vi "GINKGO - MTMP - 20180214B.vi"() -> ()   [LabVIEW 2015]
uses:
  <vilib>/rvi/interface/nirviMethod/nirviMethod.xnode
  <vilib>/rvi/interface/nirviCloseFPGA/nirviCloseFPGA.xnode
  <vilib>/rvi/interface/nirviReadWriteControl/nirviReadWriteControl.xnode
  <vilib>/rvi/interface/nirviOpenFPGA/nirviOpenFPGA.xnode
  <vilib>/rvi/interface/Simulation/niFpgaSimulationCallBeginRW.vi
  <vilib>/rvi/errors/niLvFpgaAdjustHostInterfaceError.vi
  <vilib>/rvi/errors/niLvFpgaMergeErrorWithErrorCode.vi
  <vilib>/FPGAPlugInAG/Dynamic/niLvFpga_Abort_Dynamic.vi
  <vilib>/FPGAPlugInAG/Dynamic/niLvFpga_Reset_Dynamic.vi
  <vilib>/FPGAPlugInAG/Dynamic/niLvFpga_Run_Dynamic.vi
  NiFpgaLv.dll
  <vilib>/Utility/error.llb/Error Cluster From Error Code.vi
  <vilib>/FPGAPlugInAG/Dynamic/niLvFpga_Close_Dynamic.vi
  <vilib>/FPGAPlugInAG/Dynamic/niLvFpga_ReadFifo_Dynamic.vi
  <vilib>/rvi/interface/common/dynamic/niFpgaDynamicAddResources.vi
  <vilib>/FPGAPlugInAG/Dynamic/niLvFpga_StopFifo_Dynamic.vi
  Controls/Save picture camera.vi
  <vilib>/vision/NI_Vision_Development_Module.lvlib
  Global Variable/GV_Z axis.vi
  Global Variable/GV_Lock State.vi
  <vilib>/FPGAPlugInAG/Dynamic/niLvFpga_WriteFifo_Dynamic.vi
  <vilib>/FPGAPlugInAG/Dynamic/niLvFpga_ConfigureFifo_Dynamic.vi
  <vilib>/FPGAPlugInAG/Dynamic/niLvFpga_StartFifo_Dynamic.vi
  FPGA Bitfiles/GINKGO-MTPM_7854R_FPGAControl5_d88-Mrxru6Q.lvbitx
  FPGA/FPGA Control.vi
  <vilib>/FPGAPlugInAG/PXI-7854R/niLvFpga_Open_PXI-7854R.vi
  FPGA Bitfiles/GINKGO-MTPM_7975R_FPGA796xR_a2zTekeNlbw.lvbitx
  FPGA/FPGA 796xR.vi
  <vilib>/FPGAPlugInAG/PXIe-7975R/niLvFpga_Open_PXIe-7975R.vi
  FPGA Bitfiles/GINKGO-MTPM_7853R_FPGAControl5_UMX-AIE6YDk.lvbitx
  <vilib>/FPGAPlugInAG/PXI-7853R/niLvFpga_Open_PXI-7853R.vi
  FPGA Bitfiles/GINKGO-MTPM_7961R_FPGA796xR2_HwVDrqHPH4U.lvbitx
  <vilib>/FPGAPlugInAG/PXIe-7961R/niLvFpga_Open_PXIe-7961R.vi
panel:
  out "波形图表":sgl(graph)=113.25391
  in  "ROI Statistic":bool=TRUE
  out "Mean Value":sgl=113.25391
  out "Variation":sgl=54.35391
  out "Minimal":sgl=32720.0
  out "Maximal":sgl=33176.0
  out "Power Stop":bool=TRUE
  in  "Rolling Queue Flag":bool=TRUE
  out "Total Data Out":u16=13612
  in  "Acq. Start":u16=38 caption="Phase" max=6000 step=1
  in  "Real Back Period":u16=5 min=1
  out "实际深度":u32=8388608
  in  "Map Max.":i32=10000 caption="Max."
  in  "Map Min.":i32=-500 caption="Min."
  out "Scale Value":dbl=0.1 caption="X"
  out "Total Frames":u16=16553
  in  "Max. Min.":cluster{i32, i32}(slide)={429, -176} scale=-500.0..10000.0
  in  "16-bit Display Method":u32(ring)=14 caption="Display Method" items=["Full Dynamic"=12, "Given Range"=14]
  in  "Rolling Average":dbl=2.0 min=1.0 step=1.0
  in  "Rolling":bool=TRUE
  out "User Define Phase":u32=746
  out "Image":T1(plugin-control)
  in  "Controls":T2(tab)
  in  "Start Device":bool
  in  "PMT Shutter Pow.":bool
  out "Overload Dis.":bool=TRUE
  in  "Pulse Number":enum16{"SP", "DP"}(ring)
  in  "Mems Enable":bool
  out "中心偏移":i32
  in  "互相关点数":i32=5
  in  "Calculate Phase shift":bool
  in  "Wave":enum16{"Triangle", "Sine", "Ramp"}(ring)=enum."Sine"
  in  "Interval Dis.":sgl=0.00049965957 min=-10 max=50 format="%.4f"
  in  "stop z stage":bool
  in  "5V":bool
  in  "Voltage Level":dbl=15.0 format="%#.3p"
  in  "Voltage Level 2":dbl=-15.0 caption="Voltage Level" format="%#.3p"
  in  "Source:Output Enabled":bool
  out "Voltage Measurement 2":dbl=-0.0001217159676001422 caption="Voltage Measurement"
  out "Compliance/Limit Reached 2":bool caption="Compliance/Limit Reached"
  out "Voltage Measurement":i8
  out "Compliance/Limit Reached":bool
  in  "MEMS SLOW":dbl(slide)=240000.0 caption="Slow" min=0.0 max=1000000.0 step=100.0 scale=0.0..300000.0 scale format="%#_6p"
  in  "MEMS FAST":dbl(slide) caption="Fast" min=0.0 max=1000000.0 step=100.0 scale=0.0..300000.0 scale format="%#_6p"
  out "Stimulate Time Dis.":u32
  in  "Stimulate Value":dbl=5.0 min=-10.0 max=10.0 format="%#_3f"
  in  "Stimulate Time":u32=500
  out "Stimulate Interval Time":dbl=1.9692307692307693
  in  "Stimulate Interval":u32=10
  in  "Stimulate Enable":bool caption="V.S."
  out "Frame Befor Time":dbl=845778175.0153847
  out "Frame Number":u32=4294967295
  in  "Frames Befor Stimulate":u32
  out "Acq. Sample Rate":dbl=120000000.0 caption="Sanple Rate Divider" format="%#_6p"
  in  "Microscope":enum16{"Miniature", "Benchtop"}(ring)
  in  "Line":u32(ring)=512 caption="Y" items=["8"=8, "16"=16, "32"=32, "64"=64, "128"=128, "256"=256, "512"=512, "1024"=1024, "2048"=2048]
  in  "X Offset":dbl caption="X" format="%#_3f"
  in  "Y Offset":dbl caption="Y" min=-10.0 max=10.0 format="%#_3f"
  in  "X Frequency":dbl(slide)=2600.0 caption="Speed" min=50.0 max=10000.0 step=1.0 scale=0.0..5000.0
  in  "Laser Intensity":dbl(slide)=2.0786516853932584 max=10.0 scale=0.0..5.0
  in  "Phase Shift":u32(slide)=752 caption="Phase" max=15000 step=2 scale=0.0..15000.0
  in  "Point":bool
  in  "PMT1 Sensitivity":dbl(slide)=0.5 min=0.0 max=0.95 step=0.05 scale=0.0..0.95 scale format="%#_3f"
  in  "PMT1 Enable":bool=TRUE
  out "Pixel Dwell":dbl=0.2988 format="%#_3g"
  out "Actual Positon":sgl=11.119017
  out "Actual Laser Intensity":dbl(knob)=0.69488525390625 scale=-10.0..1.0
  in  "PMT2 Switch":bool
  in  "PMT2 Sensitivity":dbl(slide)=0.45 min=0.0 max=0.95 step=0.05 scale=0.0..0.95 scale format="%#_3f"
  in  "File Name":string
  in  "Scale":bool
  in  "XY Home":bool
  in  "XY UP":bool
  in  "XY DOWN":bool
  in  "XY LEFT":bool
  in  "XY RIGHT":bool
  in  "Stop":bool=TRUE
  in  "LIVE":bool
  in  "Save":bool
  in  "Z-Stack":bool
  in  "Pixel/Line":u16(ring)=512 caption="X" items=["8"=8, "16"=16, "32"=32, "64"=64, "128"=128, "256"=256, "512"=512, "1024"=1024, "2048"=2048]
  in  "Gain":enum16{"0dB", "6dB", "12dB"}(ring)
  in  "Coulple":enum16{"AC", "DC"}(ring)=enum."DC"
  in  "Path":path=path "C:/Users/TVS001/Desktop/DATA/20180207/13-zz-gcamp" caption="Images Folder"
  out "Save Frames Dis.":u16=1000
  in  "Save Frames":u16=1000
  in  "ZOOM":u16(ring)=2 items=["User Define", "1X", "1.5X", "2X", "2.5X", "3X", "3.5X", "4X", "4.5X", "5X", "6X"]
  in  "Scan Mode":enum16{"Normal", "Line Scan", "Random Access"}(ring)
  in  "Y Amplitude":dbl=0.6 caption="Y" min=-10.0 max=18.0 format="%0.2p"
  in  "X Amplitude":dbl=0.6 caption="X" min=-10.0 max=18.0 format="%.2p"
  in  "Add Phase":bool
  in  "Move":bool=TRUE
  out "Frame Rate":dbl=5.078125 format="%#_3g"
  out "Ready":u8(slide)=10 scale=0.0..10.0
  in  "Z":bool
  out "Position":sgl=-5.9652176 format="%#_6f"
  in  "Set Zero":bool caption="空白按钮"
  in  "Reset Zero":bool caption="空白按钮"
  in  "Home Z":bool
  in  "Abs. Go":bool
  in  "Abs Pos X":sgl min=-10 max=360 format="%.6f"
  in  "Z Up":bool
  in  "Z Down":bool
  in  "Jog":sgl=0.0005 caption="Z" min=0 max=50 step=0.0001 format="%.4f"
  in  "Frames/Slice":u16=5
  in  "Slices":u16=87
  out "End Dis.":sgl=0.043470383 format="%#_6f"
  out "Start Dis.":sgl format="%#_6f"
  in  "End":bool
  in  "Start":bool
  in  "Restart":bool
  in  "Interval Time":u32=150
  in  "Zoom Standard":dbl[][](array[numeric])=[[10.0, 10.0, 11251.0], [6.66, 6.66, 10603.0], [5.0, 5.0, 10394.0], [4.0, 4.0, 10394.0], [3.34, 3.34, 8602.0], [2.86, 2.86, 10394.0], [2.5, 2.5, 10394.0], [2.222, 2.222, 10394.0], [1.3, 1.3, 8294.0], [0.6, 0.6, 8296.0]]
  in  "Zoom Miniature":dbl[][](array[numeric])=[[14.0, 8.0, 738.0], [12.0, 7.0, 746.0], [9.0, 6.0, 752.0], [7.2, 5.6, 754.0], [5.0, 4.0, 738.0], [5.14, 4.0, 846.0], [4.0, 3.0, 744.0], [3.6, 2.0, 840.0], [3.2, 2.3, 754.0], [3.0, 2.33, 740.0]]
  out "Test Point2":u32
  out "Test Point 3":u32=143394
  out "Test Point":u32
  out "Point/Pixel":i32=36
  in  "Focus Flag":bool
  out "Queue Number":i32=2
  out "Initial Z":bool
  out "Initialization Done":bool=TRUE
  in  "Start Control":bool
  out "Memory":i32(slide) scale=0.0..5000.0
  in  "Resource Name":refnum<k15>="PXI1Slot6"
  in  "Channel Name":string="1" caption="Channel Name 1"
  in  "Current Limit":dbl=0.5 format="%.3p"
  in  "Voltage Level Range":dbl=20.0 format="%.5p"
  in  "Current Limit Range":dbl=1.0 format="%.3p"
  in  "Source Delay (Sec)":dbl=0.1 format="%.3p"
  in  "Channel Name 2":string="2"
  out "Current Measurement 2":dbl=-3.1048749529460624e-06 caption="Current Measurement"
  out "Current Measurement":i16
  out "Actual DDS Ticks":u32=1
  out "Actual DDS Sample Freq":u32=279173
  in  "OUTPUT Value Ticks":u32=44
  in  "DDS Ticks":u32=1
  out "Actual OUTPUT Value Ticks":u32=44
  in  "Random 1D Array":fxp<+/-,32,16>[](array[numeric]) format="%.21g"
  in  "MG17Motor Z":refnum<k7>(container)
  out "Acq. Point Dis.":u16=32
  in  "Divide":enum16{"120M", "60M", "30M", "15M", "7.5M"}(ring)
  out "Nonlinear Acq.":bool=TRUE
  in  "Adapter Module User Data 1":u8
  in  "Adapter Module User Data 0":u8
  in  "Adapter Module User Command":u8=3
  in  "Apply":bool
  in  "HWSerialNum":i32=49871607
  in  "Set Large Scale":dbl=0.5 caption="X"
  in  "Set Small Scale":dbl=0.1 caption="X"
  in  "Set Zero Value":sgl format="%#_6f"
  in  "Fill Fraction":dbl=0.8 min=0.1 max=6.0 step=0.01
  in  "Back Period":u16=5 min=1
  in  "Initial Benchtop Speed":dbl=500.0 caption="Speed" min=50.0 max=10000.0 step=1.0
  in  "Initial Miniature Speed":dbl=2600.0 caption="Speed" min=50.0 max=10000.0 step=1.0
  out "Acq.Point Array":u16[](graph)=[38, 38, 38, 37, 37, 37, 37, 36, 36, 36, 36, 36, 35, 35, 35, 35, 35, 34, 34, 34, 34, 34, 34, 33, 33, 33, 33, 33, 33, 32, 32, 32, 32, 32, 32, 32, 32, 31, 31, 31, 31, 31, 31, 31, 31, 30, 30, 30, 30, 30, 30, 30, 30, 30, 30, 29, 29, 29, 29, 29, 29, 29, 29, 29, 29, 29, 28, 28, 28, 28, 28, 28, 28, 28, 28, 28, 28, 28, 28, 28, 27, 27, 27, 27, 27, 27, 27, 27, 27, 27, 27, 27, 27, 27, 27, 27, 26, 26, 26, 26, 26, 26, 26, 26, 26, 26, 26, 26, 26, 26, 26, 26, 26, 26, 26, 26, 26, 25, 25, 25, 25, 25, 25, 25, 25, 25, 25, 25, 25, 25, 25, 25, 25, 25, 25, 25, 25, 25, 25, 25, 25, 25, 25, 25, 24, 24, 24, 24, 24, 24, 24, 24, 24, 24, 24, 24, 24, 24, 24, 24, 24, 24, 24, 24, 24, 24, 24, 24, 24, 24, 24, 24, 24, 24, 24, 24, 24, 24, 24, 24, 24, 24, 24, 24, 24, 24, 24, 23, 23, 23, 23, 23, 23, 23, 23, 23, 23, 23, 23, 23, 23, 23, 23, 23, 23, 23, 23, 23, 23, 23, 23, 23, 23, 23, 23, 23, 23, 23, 23, 23, 23, 23, 23, 23, 23, 23, 23, 23, 23, 23, 23, 23, 23, 23, 23, 23, 23, 23, 23, 23, 23, 23, 23, 23, 23, 23, 23, 23, 23, 23, 23, 23, 23, 23, 23, 23, 23, 23, 23, 23, 23, 23, 23, 23, 23, 23, 23, 23, 23, 23, 23, 23, 23, 23, 23, 23, 23, 23, 23, 23, 23, 23, 23, 23, 23, 23, 23, 23, 23, 23, 23, 23, 23, 23, 23, 23, 23, 23, 23, 23, 23, 23, 23, 23, 23, 23, 23, 23, 23, 23, 23, 23, 23, 23, 23, 23, 23, 23, 23, 23, 23, 23, 23, 23, 23, 24, 24, 24, 24, 24, 24, 24, 24, 24, 24, 24, 24, 24, 24, 24, 24, 24, 24, 24, 24, 24, 24, 24, 24, 24, 24, 24, 24, 24, 24, 24, 24, 24, 24, 24, 24, 24, 24, 24, 24, 24, 24, 24, 25, 25, 25, 25, 25, 25, 25, 25, 25, 25, 25, 25, 25, 25, 25, 25, 25, 25, 25, 25, 25, 25, 25, 25, 25, 25, 25, 26, 26, 26, 26, 26, 26, 26, 26, 26, 26, 26, 26, 26, 26, 26, 26, 26, 26, 26, 26, 26, 27, 27, 27, 27, 27, 27, 27, 27, 27, 27, 27, 27, 27, 27, 27, 27, 28, 28, 28, 28, 28, 28, 28, 28, 28, 28, 28, 28, 28, 28, 29, 29, 29, 29, 29, 29, 29, 29, 29, 29, 29, 30, 30, 30, 30, 30, 30, 30, 30, 30, 30, 31, 31, 31, 31, 31, 31, 31, 31, 32, 32, 32, 32, 32, 32, 32, 32, 33, 33, 33, 33, 33, 33, 34, 34, 34, 34, 34, 34, 35, 35, 35, 35, 35, 36, 36, 36, 36, 36, 37, 37, 37, 37, 38, 38, 38]
  out "Init Data Out":u16[](array[numeric])=[38, 38, 38, 37, 37, 37, 37, 36, 36, 36, 36, 36, 35, 35, 35, 35, 35, 34, 34, 34, 34, 34, 34, 33, 33, 33, 33, 33, 33, 32, 32, 32, 32, 32, 32, 32, 32, 31, 31, 31, 31, 31, 31, 31, 31, 30, 30, 30, 30, 30, 30, 30, 30, 30, 30, 29, 29, 29, 29, 29, 29, 29, 29, 29, 29, 29, 28, 28, 28, 28, 28, 28, 28, 28, 28, 28, 28, 28, 28, 28, 27, 27, 27, 27, 27, 27, 27, 27, 27, 27, 27, 27, 27, 27, 27, 27, 26, 26, 26, 26, 26, 26, 26, 26, 26, 26, 26, 26, 26, 26, 26, 26, 26, 26, 26, 26, 26, 25, 25, 25, 25, 25, 25, 25, 25, 25, 25, 25, 25, 25, 25, 25, 25, 25, 25, 25, 25, 25, 25, 25, 25, 25, 25, 25, 24, 24, 24, 24, 24, 24, 24, 24, 24, 24, 24, 24, 24, 24, 24, 24, 24, 24, 24, 24, 24, 24, 24, 24, 24, 24, 24, 24, 24, 24, 24, 24, 24, 24, 24, 24, 24, 24, 24, 24, 24, 24, 24, 23, 23, 23, 23, 23, 23, 23, 23, 23, 23, 23, 23, 23, 23, 23, 23, 23, 23, 23, 23, 23, 23, 23, 23, 23, 23, 23, 23, 23, 23, 23, 23, 23, 23, 23, 23, 23, 23, 23, 23, 23, 23, 23, 23, 23, 23, 23, 23, 23, 23, 23, 23, 23, 23, 23, 23, 23, 23, 23, 23, 23, 23, 23, 23, 23, 23, 23, 23, 23, 23, 23, 23, 23, 23, 23, 23, 23, 23, 23, 23, 23, 23, 23, 23, 23, 23, 23, 23, 23, 23, 23, 23, 23, 23, 23, 23, 23, 23, 23, 23, 23, 23, 23, 23, 23, 23, 23, 23, 23, 23, 23, 23, 23, 23, 23, 23, 23, 23, 23, 23, 23, 23, 23, 23, 23, 23, 23, 23, 23, 23, 23, 23, 23, 23, 23, 23, 23, 23, 24, 24, 24, 24, 24, 24, 24, 24, 24, 24, 24, 24, 24, 24, 24, 24, 24, 24, 24, 24, 24, 24, 24, 24, 24, 24, 24, 24, 24, 24, 24, 24, 24, 24, 24, 24, 24, 24, 24, 24, 24, 24, 24, 25, 25, 25, 25, 25, 25, 25, 25, 25, 25, 25, 25, 25, 25, 25, 25, 25, 25, 25, 25, 25, 25, 25, 25, 25, 25, 25, 26, 26, 26, 26, 26, 26, 26, 26, 26, 26, 26, 26, 26, 26, 26, 26, 26, 26, 26, 26, 26, 27, 27, 27, 27, 27, 27, 27, 27, 27, 27, 27, 27, 27, 27, 27, 27, 28, 28, 28, 28, 28, 28, 28, 28, 28, 28, 28, 28, 28, 28, 29, 29, 29, 29, 29, 29, 29, 29, 29, 29, 29, 30, 30, 30, 30, 30, 30, 30, 30, 30, 30, 31, 31, 31, 31, 31, 31, 31, 31, 32, 32, 32, 32, 32, 32, 32, 32, 33, 33, 33, 33, 33, 33, 34, 34, 34, 34, 34, 34, 35, 35, 35, 35, 35, 36, 36, 36, 36, 36, 37, 37, 37, 37, 38, 38, 38]
  out "x amp. new":dbl
  out "y amp. new":dbl
  in  "Add Random Access":bool
  out "x offset new":i16=-7638
  out "y offset new":i16=-4030
  in  "All Random Array":fxp<+/-,32,16>[][](array[numeric])
  in  "Clear Array":bool
  out "Random Phase":u32=12 caption="Phase" max=6000 step=1
  # "File Name"
  # "File Path"
  # "Save Frames"
  # "Microscope"
  # "Scan Mode"
  # "PMT1"
  # "PMT2"
  # "Frame Size"
  # "Gain"
  # "Scan Speed"
  # "Hz"
  # "V"
  # "V"
  # "Rate"
  # "Frame Rate"
  # "μs"
  # "Hz"
  # "Pixel Dwell"
  # "XY"
  # "Z"
  # "Zoom"
  # "Point"
  # "Amplitude"
  # "V"
  # "V"
  # "Phase"
  # "Laser"
  # "Intensity Map"
  # "Recent Z"
  # "Frames Before"
  # "s"
  # "Stimulate Interval"
  # "s"
  # "ms"
  # "Stimulate Time"
  # "V"
  # "Stimulate Intensity"
  # "Mode Switch"
  # "MEMS Filter"
  # "Acquisition Mode"
  # "Image Settings"
  # "Magnification"
  # "Save Settings"
  # "Position Settings"
  # "Detection Settings"
  # "Z-scan Settings"
  # "Vision Stimulate Settings"
  # "X"
  # "Y"
  # "Phase"
  # "1X"
  # "1.5X"
  # "2X"
  # "2.5X"
  # "3X"
  # "3.5X"
  # "4X"
  # "4.5X"
  # "5X"
  # "6X"
  # "X"
  # "Y"
  # "Phase"
  # "1X"
  # "1.5X"
  # "2X"
  # "2.5X"
  # "3X"
  # "3.5X"
  # "4X"
  # "4.5X"
  # "5X"
  # "6X"
  # "40859011"
  # "83856379"
  # "AO0 -- X-Miniature  \nAO1 -- Y-Miniature\nAO2 -- Laser Intensity\nAO3 -- PMT1\nAO4 -- PMT2 \nAO5 -- \nAO6 -- X-Benchtop\nAO7 -- Y-Benchtop\n\nAI0  -- Actual Laser Intensity"
  # "DIO0 -- Acqusition  \nDIO1 -- VSYNC\nDIO2 -- HSYNC \nDIO3 -- Laser Shutter\nDIO4 -- MEMS FAST Filter\nDIO5 -- MEMS SLOW Filter\nDIO6 -- PMT Shutter\nDIO7 -- PMT Shutter Pow.\nDIO8 -- Shock Detection \nDIO9 -- Foot-plate LIVE Detection"
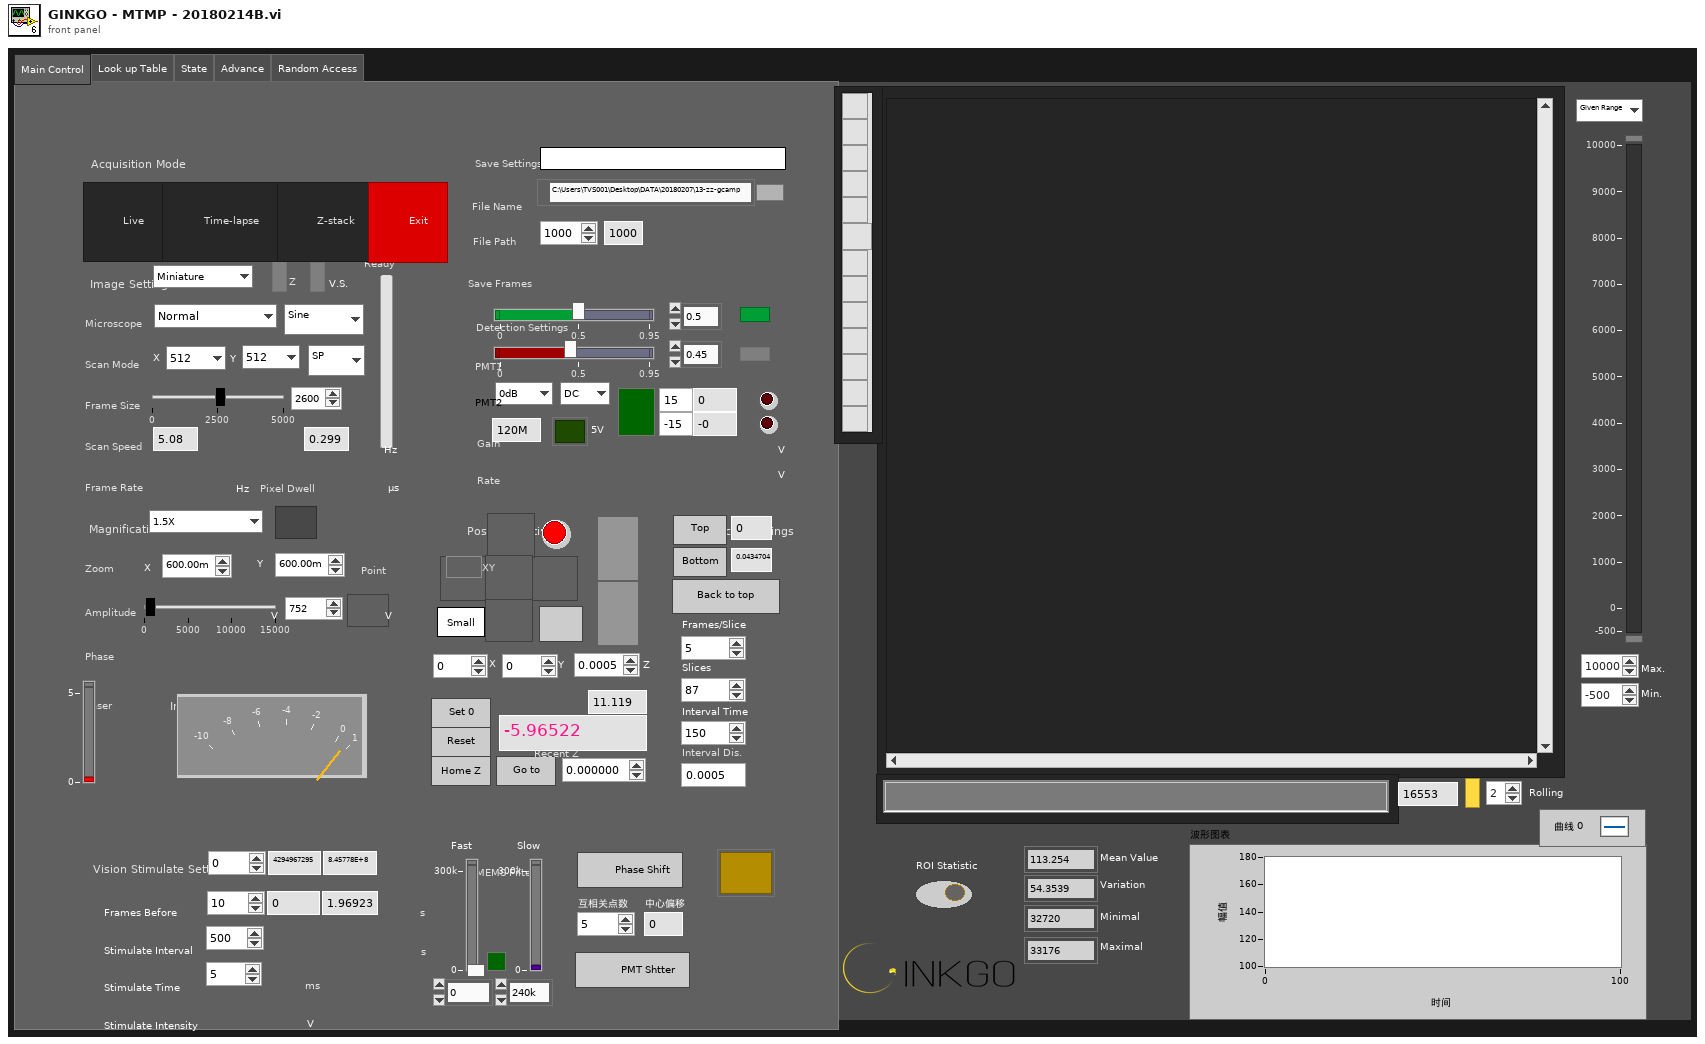
[diagram p1: front panel]
types:
  T1 = typedef "IMAQ Image.ctl" = refnum<image>
  T2 = enum32{"Main Control", "Look up Table", "State", "Advance", "Random Access"}
  T3 = typedef "Image Type" = u32
  T4 = enum8{"Enabled", "Disabled", "Disabled and Grayed Out"}
  T5 = cluster{"Global Rectangle":i32[], "Contours":cluster{"Contour Type":u32, "ROI Type":u32, "Points":i32[]}[]}
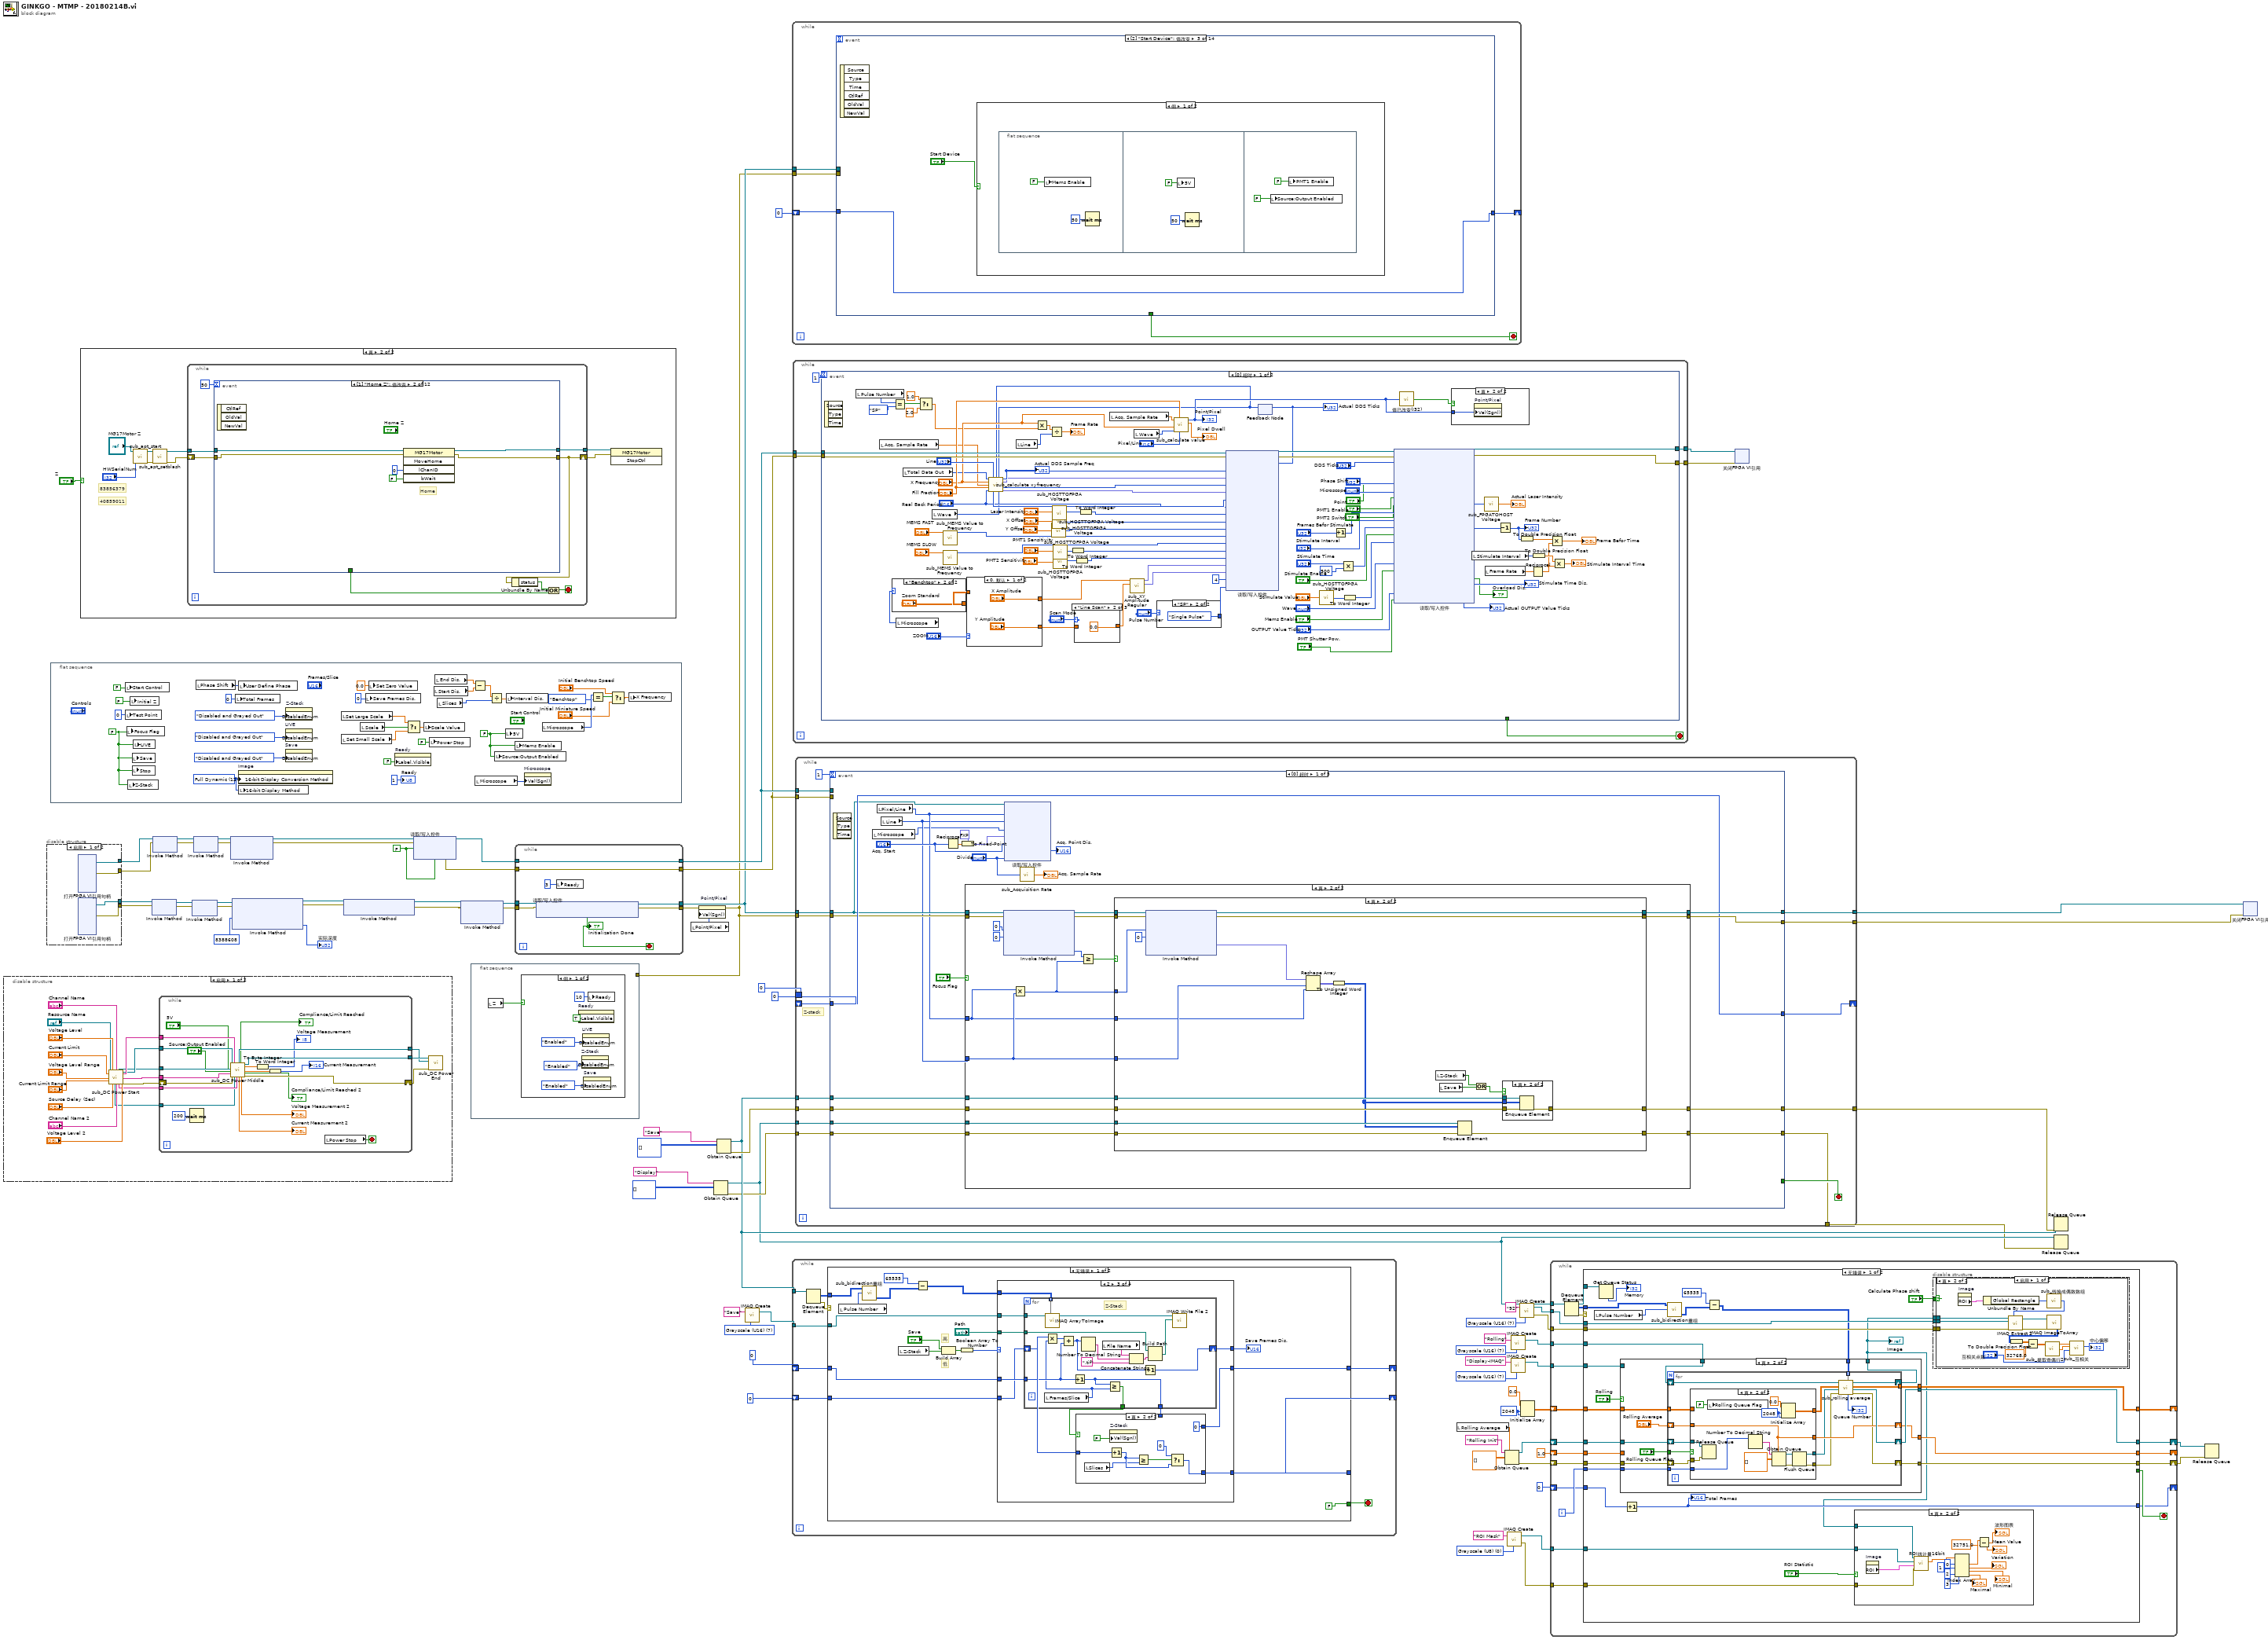
[diagram p0: block diagram]
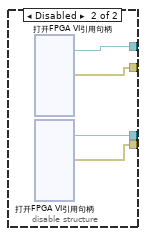
[diagram p2: hidden frame]
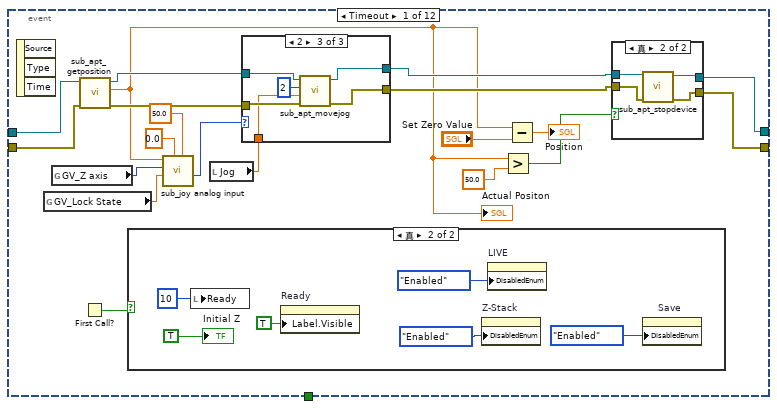
[diagram p4: hidden frame]
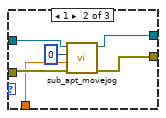
[diagram p6: hidden frame]
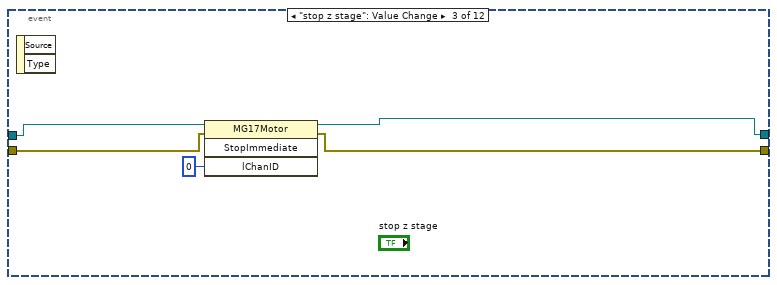
[diagram p9: hidden frame]
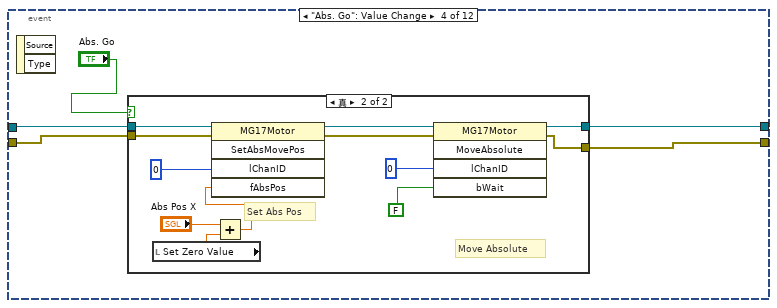
[diagram p10: hidden frame]
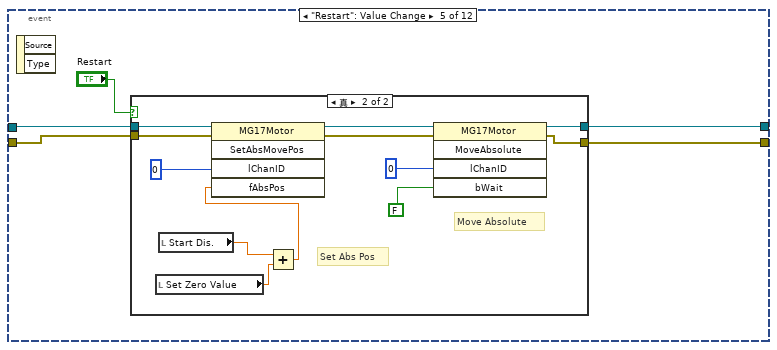
[diagram p12: hidden frame]
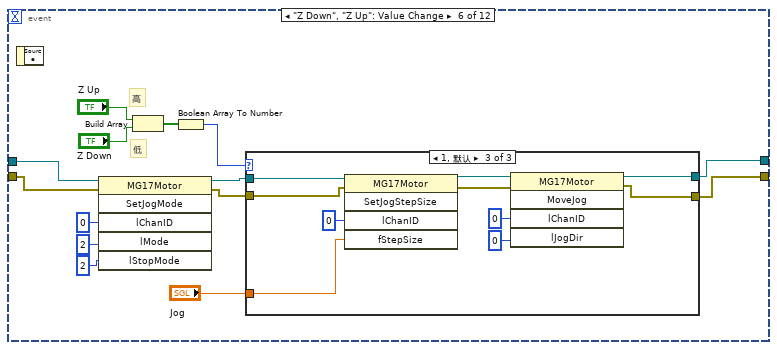
[diagram p14: hidden frame]
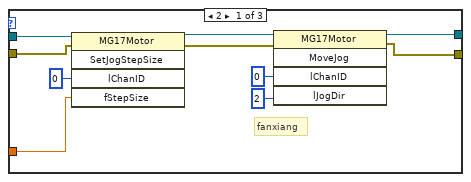
[diagram p15: hidden frame]
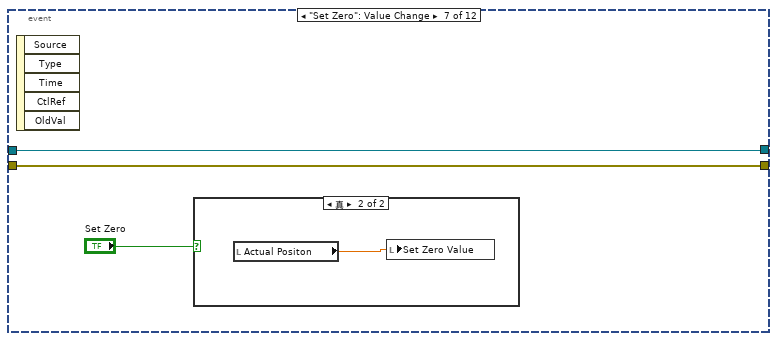
[diagram p17: hidden frame]
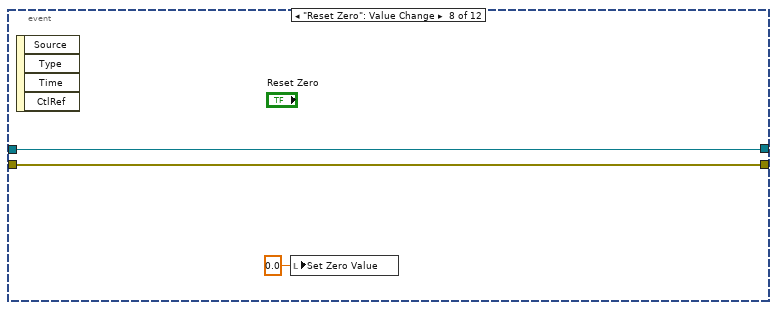
[diagram p19: hidden frame]
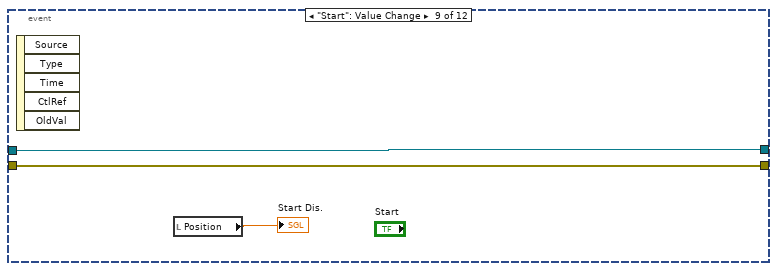
[diagram p20: hidden frame]
diagram:
  w3 = T3 0 items=["Grayscale (U8)", "Grayscale (I16)", "Grayscale (SGL)", "Complex (CSG)", "RGB (U32)", "HSL (U32)", "RGB (U64)", "Grayscale (U16)"] ("Image Type")
  w9 = T3 7 items=["Grayscale (U8)", "Grayscale (I16)", "Grayscale (SGL)", "Complex (CSG)", "RGB (U32)", "HSL (U32)", "RGB (U64)", "Grayscale (U16)"] ("Image Type")
  w15 = T3 7 items=["Grayscale (U8)", "Grayscale (I16)", "Grayscale (SGL)", "Complex (CSG)", "RGB (U32)", "HSL (U32)", "RGB (U64)", "Grayscale (U16)"] ("Image Type")
  w28 = T3 7 items=["Grayscale (U8)", "Grayscale (I16)", "Grayscale (SGL)", "Complex (CSG)", "RGB (U32)", "HSL (U32)", "RGB (U64)", "Grayscale (U16)"] ("Image Type")
  w38 = 2048 ("维数大小")
  w35 = T3 7 items=["Grayscale (U8)", "Grayscale (I16)", "Grayscale (SGL)", "Complex (CSG)", "RGB (U32)", "HSL (U32)", "RGB (U64)", "Grayscale (U16)"] ("Image Type")
  w49 = FALSE ("Enable")
  n1 = disable-structure shown="启用" {
    frame Enabled {
      n2 = call "sub_DC Power Start.vi"("IVI引用句柄输入"="Resource Name", "Current Limit"="Current Limit", "Voltage Level Range"="Voltage Level Range", "Current Limit Range"="Current Limit Range", "Voltage Level"="Voltage Level", "Source Delay (Sec)"="Source Delay (Sec)", "Channel Name"="Channel Name", "Channel Name 2"="Channel Name 2", "Voltage Level 2"="Voltage Level 2") -> ("instrument handle out 2"=w81:refnum<k15>, "instrument handle out"=w88:refnum<k15>, "Channel Name 6"=w82:string, "IVI引用句柄输出"=w96:refnum<k15>, "Channel Name 4"=w97:string, "Channel Name 3"=w90:string, "错误输出"=w87:errorcluster)  [unwired: 4 in]
      n3 = while {
        tunnel: w97 -> [w121]
        tunnel: w90 -> [w120]
        tunnel: [w119] -> w89
        shift-right: [w118] -> w86
        shift-left: w87 -> [w115]
        tunnel: w88 -> [w114]
        tunnel: w96 -> [w116]
        tunnel: [w117] -> w98
        tunnel: w82 -> [w104]
        tunnel: w81 -> [w103]
        stop <- w105 stop-if-true
        n4 = Wait (ms)(milliseconds to wait=u32 200 ("等待时间（毫秒）")) -> ()  [unwired: 1 out]
        n5 = call "sub_DC Power Middle.vi"("IVI引用句柄输入"=w116, "instrument handle out"=w114, "5V"="5V", "Source:Output Enabled"="Source:Output Enabled", "Channel Name 3"=w120, "错误输入（无错误）"=w115, "Channel Name 4"=w121, "instrument handle out 2"=w103, "Channel Name 5"=w104) -> ("instrument handle out 3"=w119:refnum<k15>, "Current Measurement 2"=→"Current Measurement 2":dbl, "Compliance/Limit Reached"=→"Compliance/Limit Reached":bool, "Voltage Measurement 2"=→"Voltage Measurement 2":dbl, "IVI引用句柄输出"=w117:refnum<k15>, "Voltage Measurement"=w111:dbl, "Current Measurement"=w110:dbl, "Compliance/Limit Reached 2"=→"Compliance/Limit Reached 2":bool, "错误输出"=w118:errorcluster)  [unwired: 2 in]
        n6 = To Byte Integer(number=w111) -> (8bit integer=→"Voltage Measurement":i8)
        n7 = To Word Integer(number=w110) -> (16bit integer=→"Current Measurement":i16)
        n8 = local read "Power Stop"() -> (w105:bool)
      }
      n9 = call "sub_DC Power End.vi"("错误输入（无错误）"=w86, "instrument handle out"=w89, "IVI引用句柄输入"=w98) -> ()  [unwired: 9 in]
    }
    frame Disabled {
    }
  }
  n10 = disable-structure shown="启用" {
    disable-tunnel: [w125 w129] -> w80
    disable-tunnel: [w124 w128] -> w79
    disable-tunnel: [w123 w126] -> w78
    disable-tunnel: [w122 w127] -> w77
    frame Enabled {
      n11 = xnode "打开FPGA VI引用句柄"() -> ("FPGA VI引用输出"=w125:refnum<k20>, "错误输出"=w124:errorcluster)  [unwired: 2 in]
      n12 = xnode "打开FPGA VI引用句柄"() -> ("FPGA VI引用输出"=w122:refnum<k20>, "错误输出"=w123:errorcluster)  [unwired: 2 in]
    }
    frame Disabled {
      n13 = xnode "打开FPGA VI引用句柄"() -> ("FPGA VI引用输出"=w129:refnum<k20>, "错误输出"=w128:errorcluster)  [unwired: 2 in]
      n14 = xnode "打开FPGA VI引用句柄"() -> ("FPGA VI引用输出"=w127:refnum<k20>, "错误输出"=w126:errorcluster)  [unwired: 2 in]
    }
  }
  n15 = flat-sequence {
    frame #0 {
      w143 = FALSE ("Focus")
      w151 = u32 12 items=["Default"=10, "Most Significant Bits"=11, "Full Dynamic"=12, "Downshift"=13, "Given Range"=14, "90% Dynamic"=15, "Given Percent Range"=16] ("16-bit Display Mapping:Conversion Method")
      w158 = FALSE ("Focus")
      n16 = local write "Start Control"(FALSE ("Initial")) -> ()
      n17 = local write "Test Point"(u32 0 ("Test Point")) -> ()
      n18 = local write "Focus Flag"(w158) -> ()
      n19 = local write "Z-Stack"(w158) -> ()
      n20 = local write "Initial Z"(FALSE ("Initial")) -> ()
      n21 = local write "Save"(w158) -> ()
      n22 = local write "Stop"(w158) -> ()
      n23 = local write "LIVE"(w158) -> ()
      n24 = local read "Phase Shift"() -> (w144:u32)
      n25 = local write "Total Frames"(u16 0 ("Total Frames")) -> ()
      n26 = property on="Image" class="ImageControl"("16-bit Display Conversion Method"=w151) -> ()  [unwired: 2 in, 2 out]
      n27 = local write "User Define Phase"(w144) -> ()
      n28 = local write "16-bit Display Method"(w151) -> ()
      n29 = property on="LIVE" class="Bool (严格)"("DisabledEnum"=T4."Disabled and Grayed Out" ("禁用")) -> ()  [unwired: 2 in, 2 out]
      n30 = property on="Save" class="Bool (严格)"("DisabledEnum"=T4."Disabled and Grayed Out" ("禁用")) -> ()  [unwired: 2 in, 2 out]
      n31 = property on="Z-Stack" class="Bool (严格)"("DisabledEnum"=T4."Disabled and Grayed Out" ("禁用")) -> ()  [unwired: 2 in, 2 out]
      n32 = local read "Set Large Scale"() -> (w150:dbl)
      n33 = local read "Set Small Scale"() -> (w149:dbl)
      n34 = local read "Scale"() -> (w148:bool)
      n35 = local write "Save Frames Dis."(u16 0 ("Save Frames Dis.")) -> ()
      n36 = local write "Set Zero Value"(sgl 0.0 ("Set Zero Value")) -> ()
      n37 = property on="Ready" class="Slide (严格)"("Label.Visible"=FALSE ("标签.可见")) -> ()  [unwired: 2 in, 2 out]
      n38 = Select(t=w150, s=w148, f=w149) -> (s? t:f=w147:dbl)
      n39 = local write "Scale Value"(w147) -> ()
      n40 = local write "Power Stop"(FALSE ("Power Stop")) -> ()
      n41 = local read "Start Dis."() -> (w140:sgl)
      n42 = local read "End Dis."() -> (w139:sgl)
      n43 = local read "Slices"() -> (w138:u16)
      n44 = Subtract(x=w139, y=w140) -> (x-y=w141:sgl)
      n45 = local read "Microscope"() -> (w137:enum16{"Miniature", "Benchtop"})
      n46 = Divide(x=w141, y=w138) -> (x/y=w142:sgl)
      n47 = local write "Source:Output Enabled"(w143) -> ()
      n48 = local write "5V"(w143) -> ()
      n49 = local write "Interval Dis."(w142) -> ()
      n50 = local write "Mems Enable"(w143) -> ()
      n51 = property on="Microscope" class="Enum (严格)"("Val(Sgnl)"=w137) -> ()  [unwired: 2 in, 2 out]
      n52 = local read "Microscope"() -> (w135:enum16{"Miniature", "Benchtop"})
      n53 = Equal?(x=w135, y=enum16{"Miniature", "Benchtop"}."Benchtop") -> (x = y?=w134:bool)
      n54 = Select(t="Initial Benchtop Speed", s=w134, f="Initial Miniature Speed") -> (s? t:f=w132:dbl)
      n55 = local write "X Frequency"(w132) -> ()
      "Ready" <- u8 1 ("Process")
    }
  }
  n56 = case shown="真" "Z" {
    frame False {
    }
    frame True {
      # "40859011"
      # "83856379"
      n57 = call "sub_apt_start.vi"("HWSerialNum"="HWSerialNum", "引用"="MG17Motor Z") -> ("错误输出"=w166:errorcluster, "引用输出"=w167:refnum<k7>)  [unwired: 8 in]
      n58 = call "sub_apt_setblash.vi"("错误输入（无错误）"=w166, "引用"=w167) -> ("错误输出"=w164:errorcluster, "引用输出"=w165:refnum<k7>)  [unwired: 8 in]
      n59 = while {
        shift-right: [w173] -> w168
        shift-left: w164 -> [w176]
        tunnel: w165 -> [w177]
        tunnel: [w175] -> w169
        stop <- w171 stop-if-true
        n60 = event shown="[1] \"Home Z\": 值改变" {
          selector: _ -> [_ _ _ _ _ _ _ _ _ _ _ _]
          dyn-events: _ -> [_ _ _ _ _ _ _ _ _ _ _ _]
          timeout: 50 -> [_ _ _ _ _ _ _ _ _ _ _ _]
          tunnel: w177 -> [w190 w225 w233 w239 w258 w278 w311 w315 w318 w321 w324 w357]
          tunnel: w176 -> [w189 w224 w232 w238 w257 w277 w310 w314 w317 w320 w323 w356]
          tunnel: [w195 w227 w231 w237 w256 w286 w311 w315 w318 w321 w333 w357] -> w175
          tunnel: [w194 w226 w230 w236 w255 w285 w310 w314 w317 w320 w332 w356] -> w173
          tunnel: [_ _ _ _ _ _ _ _ _ _ _ TRUE ("Stop")] -> w170
          event Timeout {
            n61 = event-data() -> ()  [unwired: 1 in, 3 out]
            n62 = global read "GV_Lock State.vi" "GV_Lock State"() -> (w179:dbl)
            n63 = global read "GV_Z axis.vi" "GV_Z axis"() -> (w180:i32)
            n64 = call "sub_apt_getposition.vi"("错误输入（无错误）"=w189, "引用"=w190) -> ("错误输出"=w186:errorcluster, "GetPosition_Position"=w181:sgl, "引用输出"=w187:refnum<k7>)  [unwired: 7 in]
            "Actual Positon" <- w181
            n65 = First Call?() -> (First Call?: T/F=w193:bool)
            n66 = case shown="真" w193 {
              frame False {
              }
              frame True {
                n67 = local write "Ready"(u8 10 ("Process")) -> ()
                n68 = property on="Ready" class="Slide (严格)"("Label.Visible"=TRUE ("标签.可见")) -> ()  [unwired: 2 in, 2 out]
                n69 = property on="Z-Stack" class="Bool (严格)"("DisabledEnum"=T4."Enabled" ("禁用")) -> ()  [unwired: 2 in, 2 out]
                n70 = property on="LIVE" class="Bool (严格)"("DisabledEnum"=T4."Enabled" ("禁用")) -> ()  [unwired: 2 in, 2 out]
                n71 = property on="Save" class="Bool (严格)"("DisabledEnum"=T4."Enabled" ("禁用")) -> ()  [unwired: 2 in, 2 out]
                "Initial Z" <- TRUE ("Initial")
              }
            }
            n72 = call "sub_joy analog input.vi"("上限"=50.0 ("Displacement"), "下限"=0.0 ("Displacement"), "lock输入奇偶"=w179, "x"=w180, "Displacement"=w181) -> ("x state"=w182:i32)  [unwired: 5 in, 1 out]
            n73 = local read "Jog"() -> (w178:sgl)
            n74 = case shown="2" w182 {
              tunnel: [w199 w202 w208] -> w188
              tunnel: w187 -> [w199 w205 w211]
              tunnel: w186 -> [w198 w204 w210]
              tunnel: [w198 w203 w209] -> w185
              tunnel: w178 -> [_ w201 w207]
              frame 0, Default {
              }
              frame 1 {
                n75 = call "sub_apt_movejog.vi"("错误输入（无错误）"=w204, "Rel. Pos Y"=w201, "lJogDir"=0, "引用"=w205) -> ("error out"=w203:errorcluster, "MG17Motor Y"=w202:refnum<k7>)  [unwired: 6 in]
              }
              frame 2 {
                n76 = call "sub_apt_movejog.vi"("错误输入（无错误）"=w210, "Rel. Pos Y"=w207, "lJogDir"=2, "引用"=w211) -> ("error out"=w209:errorcluster, "MG17Motor Y"=w208:refnum<k7>)  [unwired: 6 in]
              }
            }
            n77 = Greater?(x=w181, y=sgl 50.0) -> (0:w196:bool)
            n78 = Subtract(x=w181, y="Set Zero Value") -> (x-y=→"Position":sgl)
            n79 = case shown="真" w196 {
              tunnel: w188 -> [w219 w223]
              tunnel: w185 -> [w218 w222]
              tunnel: [w219 w221] -> w195
              tunnel: [w218 w220] -> w194
              frame False {
              }
              frame True {
                n80 = call "sub_apt_stopdevice.vi"("错误输入（无错误）"=w222, "引用"=w223) -> ("错误输出"=w220:errorcluster, "引用输出"=w221:refnum<k7>)  [unwired: 8 in]
              }
            }
          }
          event "Home Z": Value Change {
            # "Home"
            n81 = event-data() -> ()  [unwired: 1 in, 3 out]
            n82 = invoke class="MG17Motor" method="MoveHome"(reference=w225, error in=w224, "lChanID"=0, "bWait"=FALSE) -> (reference out=w227:refnum<k7>, error out=w226:errorcluster)  [unwired: 1 in, 3 out]
          }
          event "stop z stage": Value Change {
            n83 = event-data() -> ()  [unwired: 1 in, 2 out]
            n84 = invoke class="MG17Motor" method="StopImmediate"(reference=w233, error in=w232, "lChanID"=0) -> (reference out=w231:refnum<k7>, error out=w230:errorcluster)  [unwired: 1 in, 2 out]
          }
          event "Abs. Go": Value Change {
            n85 = event-data() -> ()  [unwired: 1 in, 2 out]
            n86 = case shown="真" "Abs. Go" {
              tunnel: w239 -> [w241 w250]
              tunnel: w238 -> [w240 w249]
              tunnel: [w241 w246] -> w237
              tunnel: [w240 w245] -> w236
              frame False {
              }
              frame True {
                # "Set Abs Pos"
                # "Move Absolute"
                n87 = local read "Set Zero Value"() -> (w243:sgl)
                n88 = Add(x="Abs Pos X", y=w243) -> (x+y=w242:sgl)
                n89 = invoke class="MG17Motor" method="SetAbsMovePos"(reference=w250, error in=w249, "lChanID"=0, "fAbsPos"=w242) -> (reference out=w248:refnum<k7>, error out=w247:errorcluster)  [unwired: 1 in, 3 out]
                n90 = invoke class="MG17Motor" method="MoveAbsolute"(reference=w248, error in=w247, "lChanID"=0, "bWait"=FALSE) -> (reference out=w246:refnum<k7>, error out=w245:errorcluster)  [unwired: 1 in, 3 out]
              }
            }
          }
          event "Restart": Value Change {
            n91 = event-data() -> ()  [unwired: 1 in, 2 out]
            n92 = case shown="真" "Restart" {
              tunnel: w258 -> [w260 w269]
              tunnel: w257 -> [w259 w268]
              tunnel: [w260 w265] -> w256
              tunnel: [w259 w264] -> w255
              frame False {
              }
              frame True {
                # "Set Abs Pos"
                # "Move Absolute"
                n93 = local read "Set Zero Value"() -> (w263:sgl)
                n94 = local read "Start Dis."() -> (w262:sgl)
                n95 = Add(x=w262, y=w263) -> (x+y=w261:sgl)
                n96 = invoke class="MG17Motor" method="SetAbsMovePos"(reference=w269, error in=w268, "lChanID"=0, "fAbsPos"=w261) -> (reference out=w267:refnum<k7>, error out=w266:errorcluster)  [unwired: 1 in, 3 out]
                n97 = invoke class="MG17Motor" method="MoveAbsolute"(reference=w267, error in=w266, "lChanID"=0, "bWait"=FALSE) -> (reference out=w265:refnum<k7>, error out=w264:errorcluster)  [unwired: 1 in, 3 out]
              }
            }
          }
          event "Z Down", "Z Up": Value Change {
            # "低"
            # "高"
            n98 = event-data() -> ()  [unwired: 1 in, 1 out]
            n99 = invoke class="MG17Motor" method="SetJogMode"(reference=w278, error in=w277, "lChanID"=0, "lMode"=2, "lStopMode"=2) -> (reference out=w280:refnum<k7>, error out=w279:errorcluster)  [unwired: 1 in, 4 out]
            n100 = Build Array("Z Up", "Z Down") -> (w282:bool[])
            n101 = Boolean Array To Number(Boolean array=w282) -> (number=w281:u32)
            n102 = case shown="1, 默认" w281 {
              tunnel: w280 -> [w296 w298 w308]
              tunnel: [w294 w298 w306] -> w286
              tunnel: w279 -> [w291 w297 w303]
              tunnel: [w289 w297 w301] -> w285
              tunnel: "Jog" -> [w287 _ w299]
              frame 2 {
                # "fanxiang"
                n103 = invoke class="MG17Motor" method="SetJogStepSize"(reference=w296, error in=w291, "lChanID"=0, "fStepSize"=w287) -> (reference out=w295:refnum<k7>, error out=w290:errorcluster)  [unwired: 1 in, 3 out]
                n104 = invoke class="MG17Motor" method="MoveJog"(reference=w295, error in=w290, "lChanID"=0, "lJogDir"=2) -> (reference out=w294:refnum<k7>, error out=w289:errorcluster)  [unwired: 1 in, 3 out]
              }
              frame 0 {
              }
              frame 1, Default {
                n105 = invoke class="MG17Motor" method="SetJogStepSize"(reference=w308, error in=w303, "lChanID"=0, "fStepSize"=w299) -> (reference out=w307:refnum<k7>, error out=w302:errorcluster)  [unwired: 1 in, 3 out]
                n106 = invoke class="MG17Motor" method="MoveJog"(reference=w307, error in=w302, "lChanID"=0, "lJogDir"=0) -> (reference out=w306:refnum<k7>, error out=w301:errorcluster)  [unwired: 1 in, 3 out]
              }
            }
          }
          event "Set Zero": Value Change {
            n107 = event-data() -> ()  [unwired: 1 in, 5 out]
            n108 = case shown="真" "Set Zero" {
              frame False {
              }
              frame True {
                n109 = local read "Actual Positon"() -> (w312:sgl)
                n110 = local write "Set Zero Value"(w312) -> ()
              }
            }
          }
          event "Reset Zero": Value Change {
            n111 = event-data() -> ()  [unwired: 1 in, 4 out]
            n112 = local write "Set Zero Value"(sgl 0.0 ("Set Zero Value")) -> ()
          }
          event "Start": Value Change {
            n113 = event-data() -> ()  [unwired: 1 in, 5 out]
            n114 = local read "Position"() -> (→"Start Dis.":sgl)
          }
          event "End": Value Change {
            n115 = event-data() -> ()  [unwired: 1 in, 3 out]
            n116 = local read "Position"() -> (→"End Dis.":sgl)
          }
          event "Move": Value Change {
            n117 = event-data() -> ()  [unwired: 1 in, 1 out]
            n118 = invoke class="MG17Motor" method="SetJogMode"(reference=w324, error in=w323, "lChanID"=0, "lMode"=2, "lStopMode"=2) -> (reference out=w325:refnum<k7>, error out=w322:errorcluster)  [unwired: 1 in, 4 out]
            n119 = Absolute Value(x="Interval Dis.") -> (abs(x)=w329:sgl)
            n120 = Greater Than 0?(x="Interval Dis.") -> (x > 0?=w330:bool)
            n121 = case shown="假" w330 {
              tunnel: w325 -> [w345 w355]
              tunnel: [w343 w353] -> w333
              tunnel: w322 -> [w340 w350]
              tunnel: [w338 w348] -> w334
              tunnel: w329 -> [w336 w346]
              frame False {
                # "fanxiang"
                n122 = invoke class="MG17Motor" method="SetJogStepSize"(reference=w345, error in=w340, "lChanID"=0, "fStepSize"=w336) -> (reference out=w344:refnum<k7>, error out=w339:errorcluster)  [unwired: 1 in, 3 out]
                n123 = invoke class="MG17Motor" method="MoveJog"(reference=w344, error in=w339, "lChanID"=0, "lJogDir"=2) -> (reference out=w343:refnum<k7>, error out=w338:errorcluster)  [unwired: 1 in, 3 out]
              }
              frame True {
                n124 = invoke class="MG17Motor" method="SetJogStepSize"(reference=w355, error in=w350, "lChanID"=0, "fStepSize"=w346) -> (reference out=w354:refnum<k7>, error out=w349:errorcluster)  [unwired: 1 in, 3 out]
                n125 = invoke class="MG17Motor" method="MoveJog"(reference=w354, error in=w349, "lChanID"=0, "lJogDir"=0) -> (reference out=w353:refnum<k7>, error out=w348:errorcluster)  [unwired: 1 in, 3 out]
              }
            }
            n126 = property on="Z-Stack" class="Bool (严格)"(error in=w334, "Val(Sgnl)"=TRUE ("值(信号)")) -> (error out=w332:errorcluster)  [unwired: 1 in, 1 out]
          }
          event "Stop": Value Change {
            n127 = event-data() -> ()  [unwired: 1 in, 4 out]
          }
        }
        n128 = Unbundle By Name(w173) -> ("status"=w172:bool)
        n129 = Or(x=w172, y=w170) -> (x .or. y?=w171:bool)
      }
      n130 = invoke class="MG17Motor" method="StopCtrl"(reference=w169, error in=w168) -> ()  [unwired: 1 in, 3 out]
    }
  }
  n131 = xnode "Invoke Method"("FPGA VI引用输入"=w77, "错误输入"=w78) -> ("FPGA VI引用输出"=w66:refnum<k20>, "错误输出"=w67:errorcluster)
  n132 = xnode "Invoke Method"("FPGA VI引用输入"=w80, "错误输入"=w79) -> ("FPGA VI引用输出"=w63:refnum<k20>, "错误输出"=w62:errorcluster)
  n133 = xnode "Invoke Method"("FPGA VI引用输入"=w66, "错误输入"=w67) -> ("FPGA VI引用输出"=w68:refnum<k20>, "错误输出"=w69:errorcluster)
  n134 = xnode "Invoke Method"("FPGA VI引用输入"=w63, "错误输入"=w62) -> ("FPGA VI引用输出"=w61:refnum<k20>, "错误输出"=w60:errorcluster)
  n135 = xnode "Invoke Method"("FPGA VI引用输入"=w61, "错误输入"=w60) -> ("FPGA VI引用输出"=w59:refnum<k20>, "错误输出"=w58:errorcluster)  [unwired: 1 in]
  n136 = xnode "Invoke Method"("FPGA VI引用输入"=w68, "错误输入"=w69, "请求的深度"=u32 8388608) -> ("FPGA VI引用输出"=w65:refnum<k20>, "错误输出"=w64:errorcluster, "实际深度"=→"实际深度":u32)
  n137 = xnode "Invoke Method"("FPGA VI引用输入"=w65, "错误输入"=w64) -> ("FPGA VI引用输出"=w31:refnum<k20>, "错误输出"=w30:errorcluster)
  n138 = xnode "读取/写入控件"("FPGA VI引用输入"=w59, "错误输入"=w58, "Shutter"=w49, "Start Control"=w49) -> ("FPGA VI引用输出"=w51:refnum<k20>, "错误输出"=w50:errorcluster)
  n139 = xnode "Invoke Method"("FPGA VI引用输入"=w31, "错误输入"=w30) -> ("FPGA VI引用输出"=w55:refnum<k20>, "错误输出"=w54:errorcluster)  [unwired: 1 in]
  n140 = flat-sequence {
    tunnel: w5 -> [_]
    frame #0 {
      n141 = local read "Z"() -> (w359:bool)
      n142 = case shown="假" w359 {
        frame False {
          n143 = property on="Ready" class="Slide (严格)"("Label.Visible"=TRUE ("标签.可见")) -> ()  [unwired: 2 in, 2 out]
          n144 = property on="Z-Stack" class="Bool (严格)"("DisabledEnum"=T4."Enabled" ("禁用")) -> ()  [unwired: 2 in, 2 out]
          n145 = property on="LIVE" class="Bool (严格)"("DisabledEnum"=T4."Enabled" ("禁用")) -> ()  [unwired: 2 in, 2 out]
          n146 = property on="Save" class="Bool (严格)"("DisabledEnum"=T4."Enabled" ("禁用")) -> ()  [unwired: 2 in, 2 out]
          n147 = local write "Ready"(u8 10 ("Process")) -> ()
        }
        frame True {
          n148 = local write "Ready"(u8 6 ("Process")) -> ()
        }
      }
    }
  }
  n149 = while {
    tunnel: w55 -> [w373]
    tunnel: w54 -> [w372]
    tunnel: [w371] -> w19
    tunnel: [w370] -> w6
    tunnel: [w369] -> w52
    tunnel: w51 -> [w369]
    tunnel: [w368] -> w47
    tunnel: w50 -> [w368]
    stop <- w366 stop-if-true
    n150 = xnode "读取/写入控件"("FPGA VI引用输入"=w373, "错误输入"=w372) -> ("FPGA VI引用输出"=w371:refnum<k20>, "错误输出"=w370:errorcluster, "Adapter Module Initialization Done"=w366:bool)
    "Initialization Done" <- w366
    n151 = local write "Ready"(u8 3 ("Process")) -> ()
  }
  n152 = local read "Point/Pixel"() -> (w7:i32)
  n153 = property on="Point/Pixel" class="DigNum (严格)"(error in=w6, "Val(Sgnl)"=w7) -> (error out=w5:errorcluster)  [unwired: 1 in, 1 out]
  n154 = Obtain Queue(name (unnamed)="Display" ("名称（未命名）"), element data type=u16[][] []) -> (queue out=w21:refnum<queue>, error out=w22:errorcluster)  [unwired: 3 in, 1 out]
  n155 = Obtain Queue(name (unnamed)="Save" ("名称（未命名）"), element data type=u16[][] []) -> (queue out=w32:refnum<queue>, error out=w76:errorcluster)  [unwired: 3 in, 1 out]
  n156 = call "IMAQ Create"("Image Name"="Save", "Image Type"=w28) -> ("New Image"=w26:T1)  [unwired: 3 in, 1 out]
  n157 = while {
    tunnel: w32 -> [w382]
    shift-right: [w378] -> _
    shift-left: u16 0 -> [w379]
    tunnel: w26 -> [w377]
    shift-right: [w375] -> _
    shift-left: u16 0 -> [w376]
    stop <- w374 stop-if-true
    n158 = Dequeue Element(queue=w382) -> (element=w380:u16[][], error out=w381:errorcluster)  [unwired: 2 in, 2 out]
    n159 = case shown="无错误" w381 {
      tunnel: w380 -> [w385 _]
      tunnel: w379 -> [w399 w469]
      tunnel: [w398 w469] -> w378
      tunnel: w377 -> [w396 _]
      tunnel: w376 -> [w389 w468]
      tunnel: [w388 w468] -> w375
      tunnel: [FALSE TRUE] -> w374
      frame No Error {
        # "高"
        # "低"
        n160 = local read "Pulse Number"() -> (w384:enum16{"SP", "DP"})
        n161 = call "sub_bidirection重组.vi"("Pulse Number"=w384, "Input"=w385) -> ("合并数组"=w383:u16[][][])  [unwired: 1 in, 2 out]
        n162 = local read "Z-Stack"() -> (w394:bool)
        n163 = Subtract(x=u16 65535, y=w383) -> (x-y=w386:u16[][][])
        n164 = Build Array("Save", w394) -> (w393:bool[])
        n165 = Boolean Array To Number(Boolean array=w393) -> (number=w392:u32)
        n166 = case shown="2" w392 {
          tunnel: w399 -> [w401 w409 w430 w465]
          tunnel: [u16 0 w408 w432 u16 0] -> w398
          tunnel: w396 -> [_ w407 w436 _]
          tunnel: w386 -> [_ w406 w435 _]
          tunnel: "Path" -> [_ w405 w434 _]
          tunnel: [w401 w404 w428 w465] -> w390
          tunnel: w389 -> [_ _ w429 _]
          tunnel: [u16 0 ("t") u16 0 ("t") w431 u16 0] -> w388
          frame 0, Default {
          }
          frame 1 {
            n167 = for {
              tunnel: w409 -> [w423]
              tunnel: [w422] -> w408
              tunnel: w407 -> [w421]
              tunnel: w406 -> [w420] mode=indexing
              tunnel: w405 -> [w419]
              tunnel: [w418] -> w404
              # "Save"
              n168 = call "IMAQ ArrayToImage"("Image Pixels (U16)"=w420, "Image"=w421) -> ("Image Out"=w411:T1)  [unwired: 8 in, 1 out]
              n169 = Number To Decimal String(number=w423) -> (decimal integer string=w416:string)  [unwired: 1 in]
              n170 = Increment(x=w423) -> (x+1=w418:u16)
              n171 = Concatenate Strings("File Name", w416, ".tif" ("字符串")) -> (w417:string)
              n172 = Greater Or Equal?(x=w418, y="Save Frames") -> (x >= y?=w412:bool)
              n173 = case shown="真" w412 {
                tunnel: [w424 u16 0] -> w422
                tunnel: w418 -> [w424 _]
                frame False {
                }
                frame True {
                  n174 = property on="Save" class="Bool (严格)"("Val(Sgnl)"=FALSE ("Save")) -> ()  [unwired: 2 in, 2 out]
                }
              }
              n175 = Build Path(base path=w419, name or relative path=w417) -> (appended path=w414:path)
              n176 = call-poly "IMAQ Write File 2"("File Path"=w414, "Image"=w411) -> ()  [unwired: 8 in, 2 out]
            }
          }
          frame 2 {
            n177 = for {
              tunnel: w436 -> [w449]
              tunnel: w435 -> [w447] mode=indexing
              tunnel: w434 -> [w446]
              tunnel: [w445] -> w433
              tunnel: w430 -> [w443]
              tunnel: [w438] -> w427
              shift-right: [w439] -> w428
              shift-left: w429 -> [w442]
              # "Z-Stack"
              n178 = local read "Frames/Slice"() -> (w441:u16)
              n179 = call "IMAQ ArrayToImage"("Image Pixels (U16)"=w447, "Image"=w449) -> ("Image Out"=w448:T1)  [unwired: 8 in, 1 out]
              n180 = Multiply(x=w442, y=w441) -> (x*y=w444:u16)
              n181 = Add(x=w444, y=w443) -> (x+y=w440:u16)
              n182 = Increment(x=w443) -> (x+1=w445:u16)
              n183 = Number To Decimal String(number=w440) -> (decimal integer string=w452:string)  [unwired: 1 in]
              n184 = local read "File Name"() -> (w437:string)
              n185 = Greater Or Equal?(x=w445, y=w441) -> (x >= y?=w438:bool)
              n186 = Concatenate Strings(w437, w452, ".tif" ("字符串")) -> (w453:string)
              n187 = Increment(x=w440) -> (x+1=w439:u16)
              n188 = Build Path(base path=w446, name or relative path=w453) -> (appended path=w450:path)
              n189 = call-poly "IMAQ Write File 2"("File Path"=w450, "Image"=w448) -> ()  [unwired: 8 in, 2 out]
            }
            n190 = case shown="真" w427 {
              tunnel: w433 -> [w455 _]
              tunnel: w429 -> [w454 w460]
              tunnel: [w455 u16 0 ("t")] -> w432
              tunnel: [w454 w458] -> w431
              frame False {
              }
              frame True {
                n191 = local read "Slices"() -> (w456:u16)
                n192 = Increment(x=w460) -> (x+1=w457:u16)
                n193 = property on="Z-Stack" class="Bool (严格)"("Val(Sgnl)"=FALSE ("Save")) -> ()  [unwired: 2 in, 2 out]
                n194 = Greater Or Equal?(x=w457, y=w456) -> (x >= y?=w461:bool)
                n195 = Select(t=u16 0, s=w461, f=w457) -> (s? t:f=w458:u16)
              }
            }
          }
          frame 3 {
          }
        }
        "Save Frames Dis." <- w390
      }
      frame Error {
      }
    }
  }
  n196 = while {
    tunnel: w19 -> [w474]
    tunnel: w5 -> [w473]
    shift-right: [w470] -> _
    shift-left: 0 ("t") -> [w471]
    stop <- w472 stop-if-true
    n197 = event shown="[2] \"Start Device\": 值改变" {
      selector: _ -> [_ _ _ _ _ _ _ _ _ _ _ _ _ _]
      dyn-events: _ -> [_ _ _ _ _ _ _ _ _ _ _ _ _ _]
      timeout: _ -> [_ _ _ _ _ _ _ _ _ _ _ _ _ _]
      tunnel: w474 -> [_ w526 _ _ _ _ _ _ _ w647 w655 w705 _ _]
      tunnel: w473 -> [_ w524 _ _ _ _ _ _ _ w646 w654 w704 _ _]
      tunnel: [_ _ _ _ _ _ _ _ _ _ _ _ _ TRUE] -> w472
      tunnel: w471 -> [w475 w513 w530 w545 w561 w582 w587 w601 w632 w645 w652 w702 w742 _]
      tunnel: [w475 w513 w530 w545 w561 w582 w587 w601 w631 w645 w652 w702 w742 u16 0 ("t")] -> w470
      event "XY RIGHT", "XY LEFT", "XY DOWN", "XY UP", "XY Home": Value Change {
        n198 = event-data() -> ()  [unwired: 1 in, 6 out]
        n199 = Build Array("XY Home", "XY UP", "XY DOWN", "XY LEFT", "XY RIGHT") -> (w481:bool[])
        n200 = Boolean Array To Number(Boolean array=w481) -> (number=w482:u32)
        n201 = case shown="16" w482 {
          tunnel: [w486 0.0 w489 w494 w499 w503] -> w484
          tunnel: [w485 0.0 w491 w495 w497 w502] -> w483
          frame 0, Default {
            n202 = local read "X Offset"() -> (w486:dbl)
            n203 = local read "Y Offset"() -> (w485:dbl)
          }
          frame 1 {
            # "Home"
          }
          frame 2 {
            # "UP"
            n204 = local read "Scale Value"() -> (w492:dbl)
            n205 = local read "X Offset"() -> (w489:dbl)
            n206 = local read "Y Offset"() -> (w490:dbl)
            n207 = Add(x=w490, y=w492) -> (x+y=w491:dbl)
          }
          frame 4 {
            # "DOWN"
            n208 = local read "Scale Value"() -> (w496:dbl)
            n209 = local read "Y Offset"() -> (w493:dbl)
            n210 = local read "X Offset"() -> (w494:dbl)
            n211 = Subtract(x=w493, y=w496) -> (x-y=w495:dbl)
          }
          frame 8 {
            # "LEFT"
            n212 = local read "Scale Value"() -> (w500:dbl)
            n213 = local read "X Offset"() -> (w498:dbl)
            n214 = local read "Y Offset"() -> (w497:dbl)
            n215 = Add(x=w498, y=w500) -> (x+y=w499:dbl)
          }
          frame 16 {
            # "RIGHT"
            n216 = local read "Scale Value"() -> (w504:dbl)
            n217 = local read "X Offset"() -> (w501:dbl)
            n218 = local read "Y Offset"() -> (w502:dbl)
            n219 = Subtract(x=w501, y=w504) -> (x-y=w503:dbl)
          }
        }
        n220 = local write "X Offset"(w484) -> ()
        n221 = local write "Y Offset"(w483) -> ()
      }
      event "Nonlinear Acq.", "Point/Pixel", "Microscope", "Wave": Value Change {
        n222 = event-data() -> ()  [unwired: 1 in, 3 out]
        n223 = local read "Wave"() -> (w507:enum16{"Triangle", "Sine", "Ramp"})
        n224 = local read "Acq. Sample Rate"() -> (w523:dbl)
        n225 = local read "X Frequency"() -> (w521:dbl)
        n226 = local read "Fill Fraction"() -> (w522:dbl)
        n227 = local read "Pixel/Line"() -> (w520:u16)
        n228 = Equal?(x=w507, y=enum16{"Triangle", "Sine", "Ramp"}."Sine") -> (x = y?=w505:bool)
        "Nonlinear Acq." <- w505
        n229 = local read "Point/Pixel"() -> (w511:i32)
        n230 = To Double Precision Float(number=w520) -> (double precision float=w519:dbl)
        n231 = call "sub_Sin Acq Point.vi"("Nonlinear Acq."=w505, "Point/Pixel"=w511, "Effecte Pixel/Line"=w519, "Fill Fraction"=w522, "Scanning Speed"=w521, "Sample Rate"=w523) -> ("Total Data Out"=→"Total Data Out":u16, "Init Data Out"=w510:u16[], "Init Data Out FXP"=w509:fxp<+,18,0>[])  [unwired: 3 in]
        "Acq.Point Array" <- w510
        "Init Data Out" <- w510
        n232 = Index Array(array=w510, index=0 ("索引")) -> (element=w514:u16)
        n233 = local write "Acq. Start"(w514) -> ()
        n234 = xnode "Invoke Method"("FPGA VI引用输入"=w526, "错误输入"=w524, "数据"=w509, "超时(ms)"=0) -> ("FPGA VI引用输出"=w518:refnum<k20>, "错误输出"=w517:errorcluster)  [unwired: 1 out]
        n235 = local read "Microscope"() -> (w508:enum16{"Miniature", "Benchtop"})
        n236 = case shown="\"Miniature\", 默认" w508 {
          frame "Miniature", Default {
            n237 = local write "Real Back Period"("Back Period") -> ()
          }
          frame "Benchtop" {
            n238 = local write "Real Back Period"(u16 1 ("Back Period")) -> ()
          }
        }
        n239 = xnode "Invoke Method"("FPGA VI引用输入"=w518, "错误输入"=w517, "数据"=w510, "超时(ms)"=0) -> ()  [unwired: 3 out]
      }
      event "Start Device": Value Change {
        n240 = event-data() -> ()  [unwired: 1 in, 6 out]
        n241 = case shown="假" "Start Device" {
          frame False {
            n242 = flat-sequence {
              frame #0 {
                n243 = local write "Mems Enable"(FALSE ("Mems Enable")) -> ()
                n244 = Wait (ms)(milliseconds to wait=u32 50 ("等待时间（毫秒）")) -> ()  [unwired: 1 out]
              }
              frame #1 {
                n245 = local write "5V"(FALSE ("5V")) -> ()
                n246 = Wait (ms)(milliseconds to wait=u32 50 ("等待时间（毫秒）")) -> ()  [unwired: 1 out]
              }
              frame #2 {
                n247 = local write "Source:Output Enabled"(FALSE ("Source:Output Enabled")) -> ()
                n248 = local write "PMT1 Enable"(FALSE ("PMT1 Enable")) -> ()
              }
            }
          }
          frame True {
            n249 = flat-sequence {
              frame #0 {
                n250 = local write "Source:Output Enabled"(TRUE ("Source:Output Enabled")) -> ()
                n251 = local write "PMT1 Enable"(TRUE ("PMT1 Enable")) -> ()
                n252 = Wait (ms)(milliseconds to wait=u32 50 ("等待时间（毫秒）")) -> ()  [unwired: 1 out]
              }
              frame #1 {
                n253 = local write "5V"(TRUE ("5V")) -> ()
                n254 = Wait (ms)(milliseconds to wait=u32 50 ("等待时间（毫秒）")) -> ()  [unwired: 1 out]
              }
              frame #2 {
                n255 = local write "Mems Enable"(TRUE ("Mems Enable")) -> ()
              }
            }
          }
        }
      }
      event "Add Phase": Value Change {
        n256 = event-data() -> ()  [unwired: 1 in, 6 out]
        n257 = local read "Scan Mode"() -> (w544:enum16{"Normal", "Line Scan", "Random Access"})
        n258 = local read "Phase Shift"() -> (w543:u32)
        n259 = case shown="\"Normal\", 默认" w544 {
          tunnel: w543 -> [w546 w547]
          frame "Random Access" {
            "Random Phase" <- w546
          }
          frame "Normal", Default {
            n260 = local read "Microscope"() -> (w555:enum16{"Miniature", "Benchtop"})
            n261 = case shown="\"Miniature\", 默认" w555 {
              tunnel: [w558 w559] -> w554
              frame "Miniature", Default {
                n262 = local read "Zoom Miniature"() -> (w558:dbl[][])
              }
              frame "Benchtop" {
                n263 = local read "Zoom Standard"() -> (w559:dbl[][])
              }
            }
            n264 = local read "ZOOM"() -> (w553:u16)
            n265 = Decrement(x=w553) -> (x-1=w551:u16)
            n266 = Index Array(array=w554, index (row)=w551) -> (element=w548:dbl[])  [unwired: 1 in]
            n267 = Insert Into Array(array=w548, index=2 ("索引"), new element=w547) -> (w550:dbl[])
            n268 = case shown="0, 默认" w553 {
              frame 0, Default {
                n269 = local read "Phase Shift"() -> (→"User Define Phase":u32)
              }
              frame 1 {
              }
            }
            n270 = Replace Array Subset(array=w554, new element=w550, index (row)=w551) -> (w552:dbl[][])  [unwired: 1 in]
            n271 = case shown="\"Miniature\", 默认" w555 {
              tunnel: w552 -> [w556 w557]
              frame "Miniature", Default {
                n272 = local write "Zoom Miniature"(w556) -> ()
              }
              frame "Benchtop" {
                n273 = local write "Zoom Standard"(w557) -> ()
              }
            }
          }
        }
      }
      event "Scan Mode", "ZOOM": Value Change {
        n274 = event-data() -> ()  [unwired: 1 in, 6 out]
        n275 = local read "Microscope"() -> (w568:enum16{"Miniature", "Benchtop"})
        n276 = case shown="\"Miniature\", 默认" w568 {
          tunnel: [w572 w573] -> w565
          frame "Miniature", Default {
            n277 = local read "Zoom Miniature"() -> (w572:dbl[][])
          }
          frame "Benchtop" {
            n278 = local read "Zoom Standard"() -> (w573:dbl[][])
          }
        }
        n279 = local read "ZOOM"() -> (w564:u16)
        n280 = case shown="0, 默认" w564 {
          selector: w564 -> [_ w577]
          tunnel: w565 -> [_ w578]
          tunnel: [w574 w576] -> w567
          frame 0, Default {
            n281 = local read "User Define Phase"() -> (w574:u32)
          }
          frame 1..10 {
            n282 = Decrement(x=w577) -> (x-1=w580:u16)
            n283 = Index Array(array=w578, index (row)=w580) -> (element=w581:dbl[])  [unwired: 1 in]
            n284 = Index Array(array=w581, index=2 ("索引")) -> (element=w575:dbl)
            n285 = To Unsigned Long Integer(number=w575) -> (unsigned 32bit integer=w576:u32)
          }
        }
        n286 = local read "Random Phase"() -> (w566:u32)
        n287 = local read "Scan Mode"() -> (w563:enum16{"Normal", "Line Scan", "Random Access"})
        n288 = case shown="\"Normal\", 默认" w563 {
          tunnel: w567 -> [w569 w570 _]
          tunnel: w566 -> [_ _ w571]
          tunnel: [w569 w570 w571] -> w562
          frame "Normal", Default {
          }
          frame "Line Scan" {
          }
          frame "Random Access" {
          }
        }
        n289 = local write "Phase Shift"(w562) -> ()
      }
      event "Set Large Scale", "Set Small Scale", "Scale": Value Change {
        n290 = event-data() -> ()  [unwired: 1 in, 6 out]
        n291 = Select(t="Set Large Scale", s="Scale", f="Set Small Scale") -> (s? t:f=→"Scale Value":dbl)
      }
      event "16-bit Display Method", "Map Max.", "Map Min.", "Max. Min.": Value Change {
        n292 = event-data() -> ()  [unwired: 1 in, 6 out]
        n293 = local read "16-bit Display Method"() -> (w588:u32)
        n294 = Unbundle("Max. Min.") -> (w591:i32, w595:i32)
        n295 = case shown="14" w588 {
          frame 0, Default {
          }
          frame 14 {
            n296 = To Double Precision Float(number="Map Max.") -> (double precision float=w598:dbl)
            n297 = To Double Precision Float(number="Map Min.") -> (double precision float=w597:dbl)
            n298 = property on="Max. Min." class="Slide (严格)"("Scale.Maximum"=w598, "Scale.Minimum"=w597) -> ()  [unwired: 2 in, 2 out]
          }
        }
        n299 = Add(x=w595, y=32768) -> (x+y=w593:i32)
        n300 = Add(x=w591, y=32768) -> (x+y=w592:i32)
        n301 = property on="Image" class="ImageControl"("16-bit Display Conversion Method"="16-bit Display Method", "16-bit Display Maximum Value"=w592, "16-bit Display Minimum Value"=w593) -> ()  [unwired: 2 in, 2 out]
      }
      event "Image": Mouse Up {
        n302 = event-data() -> ()  [unwired: 1 in, 8 out]
        n303 = disable-structure shown="禁用" {
          frame Disabled {
            n304 = local read "Microscope"() -> (w605:enum16{"Miniature", "Benchtop"})
            n305 = case shown="\"Benchtop\"" w605 {
              tunnel: [w615 w616] -> w606
              frame "Miniature", Default {
                n306 = local read "Zoom Miniature"() -> (w615:dbl[][])
              }
              frame "Benchtop" {
                n307 = local read "Zoom Standard"() -> (w616:dbl[][])
              }
            }
            n308 = local read "ZOOM"() -> (w604:u16)
            n309 = case shown="0, 默认" w604 {
              selector: w604 -> [_ w621]
              tunnel: [w617 w619] -> w602
              tunnel: [w618 w620] -> w603
              tunnel: w606 -> [_ w622]
              frame 0, Default {
                n310 = local read "X Amplitude"() -> (w618:dbl)
                n311 = local read "Y Amplitude"() -> (w617:dbl)
              }
              frame 1..10 {
                n312 = Decrement(x=w621) -> (x-1=w625:u16)
                n313 = Index Array(array=w622, index (row)=w625) -> (element=w626:dbl[])  [unwired: 1 in]
                n314 = Index Array(array=w626, index #1=0 ("索引"), index #2=1 ("索引")) -> (element #1=w620:dbl, element #2=w619:dbl)  [unwired: 1 in, 1 out]
              }
            }
            n315 = property on="Image" class="ImageControl"() -> ("ROI"=w614:T5)  [unwired: 2 in, 2 out]
            n316 = local read "Pixel/Line"() -> (w611:u16)
            n317 = local read "Line"() -> (w610:u32)
            n318 = Unbundle By Name(w614) -> ("Global Rectangle"=w613:i32[])
            n319 = call "sub_new x y amplitude.vi"("Global Rectangle"=w613, "Line"=w610, "Pixel/Line"=w611, "y amp."=w602, "x amp."=w603) -> ("y offset new"=→"y offset new":i16, "x offset new"=→"x offset new":i16, "y amp. new"=→"y amp. new":dbl, "x amp. new"=→"x amp. new":dbl)  [unwired: 3 in]
          }
          frame Enabled {
          }
        }
      }
      event "Add Random Access", "Clear Array": Value Change {
        n320 = event-data() -> ()  [unwired: 1 in, 6 out]
        n321 = case shown="真" "Add Random Access" {
          tunnel: w632 -> [w635 w639]
          tunnel: [w635 w640] -> w629
          frame False {
          }
          frame True {
            n322 = local read "x amp. new"() -> (w644:dbl)
            n323 = local read "y amp. new"() -> (w643:dbl)
            n324 = local read "x offset new"() -> (w642:i16)
            n325 = local read "y offset new"() -> (w641:i16)
            n326 = call "sub_new amplitude to array.vi"("Index Row"=w639, "All Random Array In"="All Random Array", "y offset new"=w641, "x offset new"=w642, "y amp. new"=w643, "x amp. new"=w644) -> ("All Random Array Out"=w637:fxp<+/-,32,16>[][])  [unwired: 4 in, 1 out]
            n327 = Increment(x=w639) -> (x+1=w640:i32)
            n328 = local write "All Random Array"(w637) -> ()
            n329 = call "sub_2D Array to 1D.vi"("2D Array"=w637) -> ("Random 1D Array"=w636:fxp<+/-,32,16>[])
            n330 = local write "Random 1D Array"(w636) -> ()
          }
        }
        n331 = case shown="真" "Clear Array" {
          frame False {
          }
          frame True {
            n332 = local write "Random 1D Array"(fxp<+/-,32,16>[] [0.0, 0.0, 0.0, 0.0, 0.0, 0.0, 0.0, 0.0, 0.0, 0.0, 0.0, 0.0, 0.0, 0.0, 0.0, 0.0, 0.0, 0.0, 0.0, 0.0, 0.0, 0.0, 0.0, 0.0, 0.0, 0.0, 0.0, 0.0, 0.0, 0.0, 0.0, 0.0, 0.0, 0.0, 0.0, 0.0, 0.0, 0.0, 0.0, 0.0, 0.0, 0.0, 0.0, 0.0, 0.0, 0.0, 0.0, 0.0, 0.0, 0.0, 0.0, 0.0, 0.0, 0.0, 0.0, 0.0, 0.0, 0.0, 0.0, 0.0, 0.0, 0.0, 0.0, 0.0, 0.0, 0.0, 0.0, 0.0, 0.0, 0.0, 0.0, 0.0, 0.0, 0.0, 0.0, 0.0, 0.0, 0.0, 0.0, 0.0, 0.0, 0.0, 0.0, 0.0, 0.0, 0.0, 0.0, 0.0, 0.0, 0.0, 0.0, 0.0, 0.0, 0.0, 0.0, 0.0, 0.0, 0.0, 0.0, 0.0, 0.0, 0.0, 0.0, 0.0, 0.0, 0.0, 0.0, 0.0, 0.0, 0.0, 0.0, 0.0, 0.0, 0.0, 0.0, 0.0, 0.0, 0.0, 0.0, 0.0, 0.0, 0.0, 0.0, 0.0, 0.0, 0.0, 0.0, 0.0, 0.0, 0.0, 0.0, 0.0, 0.0, 0.0, 0.0, 0.0, 0.0, 0.0, 0.0, 0.0, 0.0, 0.0, 0.0, 0.0, 0.0, 0.0, 0.0, 0.0, 0.0, 0.0, 0.0, 0.0, 0.0, 0.0, 0.0, 0.0, 0.0, 0.0, 0.0, 0.0, 0.0, 0.0, 0.0, 0.0, 0.0, 0.0, 0.0, 0.0, 0.0, 0.0, 0.0, 0.0, 0.0, 0.0, 0.0, 0.0, 0.0, 0.0, 0.0, 0.0, 0.0, 0.0, 0.0, 0.0, 0.0, 0.0, 0.0, 0.0, 0.0, 0.0, 0.0, 0.0, 0.0, 0.0, 0.0, 0.0, 0.0, 0.0, 0.0, 0.0] ("Random 1D Array")) -> ()
            n333 = local write "All Random Array"(fxp<+/-,32,16>[][] [] ("All Random Array")) -> ()
          }
        }
        n334 = Select(t=0, s="Clear Array", f=w629) -> (s? t:f=w631:i32)
      }
      event "Apply": Value Change {
        n335 = event-data() -> ()  [unwired: 1 in, 6 out]
        n336 = xnode "读取/写入控件"("FPGA VI引用输入"=w647, "错误输入"=w646, "Adapter Module User Command"="Adapter Module User Command", "Adapter Module User Data 0"="Adapter Module User Data 0", "Adapter Module User Data 1"="Adapter Module User Data 1", "Adapter Module Do User Command Commit"="Apply") -> ()  [unwired: 2 out]
      }
      event "Gain": Value Change {
        n337 = event-data() -> ()  [unwired: 1 in, 6 out]
        n338 = local read "Microscope"() -> (w653:enum16{"Miniature", "Benchtop"})
        n339 = case shown="\"0dB\", 默认" "Gain" {
          tunnel: w655 -> [w659 w674 w689]
          tunnel: w654 -> [w658 w673 w688]
          tunnel: w653 -> [w657 w672 w687]
          frame "0dB", Default {
            n340 = case shown="\"Miniature\", 默认" w657 {
              tunnel: w659 -> [w665 w667]
              tunnel: w658 -> [w664 w666]
              frame "Miniature", Default {
                n341 = xnode "读取/写入控件"("FPGA VI引用输入"=w665, "错误输入"=w664, "Adapter Module User Command"=u8 2, "Adapter Module User Data 0"=u8 0, "Adapter Module User Data 1"=u8 0, "Adapter Module Do User Command Commit"=TRUE) -> ()  [unwired: 2 out]
              }
              frame "Benchtop" {
                n342 = xnode "读取/写入控件"("FPGA VI引用输入"=w667, "错误输入"=w666, "Adapter Module User Command"=u8 2, "Adapter Module User Data 0"=u8 1, "Adapter Module User Data 1"=u8 0, "Adapter Module Do User Command Commit"=TRUE) -> ()  [unwired: 2 out]
              }
            }
          }
          frame "6dB" {
            n343 = case shown="\"Benchtop\"" w672 {
              tunnel: w674 -> [w680 w682]
              tunnel: w673 -> [w679 w681]
              frame "Miniature", Default {
                n344 = xnode "读取/写入控件"("FPGA VI引用输入"=w680, "错误输入"=w679, "Adapter Module User Command"=u8 2, "Adapter Module User Data 0"=u8 0, "Adapter Module User Data 1"=u8 1, "Adapter Module Do User Command Commit"=TRUE) -> ()  [unwired: 2 out]
              }
              frame "Benchtop" {
                n345 = xnode "读取/写入控件"("FPGA VI引用输入"=w682, "错误输入"=w681, "Adapter Module User Command"=u8 2, "Adapter Module User Data 0"=u8 1, "Adapter Module User Data 1"=u8 1, "Adapter Module Do User Command Commit"=TRUE) -> ()  [unwired: 2 out]
              }
            }
          }
          frame "12dB" {
            n346 = case shown="\"Miniature\", 默认" w687 {
              tunnel: w689 -> [w691 w701]
              tunnel: w688 -> [w690 w700]
              frame "Miniature", Default {
                n347 = xnode "读取/写入控件"("FPGA VI引用输入"=w691, "错误输入"=w690, "Adapter Module User Command"=u8 2, "Adapter Module User Data 0"=u8 0, "Adapter Module User Data 1"=u8 2, "Adapter Module Do User Command Commit"=TRUE) -> ()  [unwired: 2 out]
              }
              frame "Benchtop" {
                n348 = xnode "读取/写入控件"("FPGA VI引用输入"=w701, "错误输入"=w700, "Adapter Module User Command"=u8 2, "Adapter Module User Data 0"=u8 1, "Adapter Module User Data 1"=u8 2, "Adapter Module Do User Command Commit"=TRUE) -> ()  [unwired: 2 out]
              }
            }
          }
        }
      }
      event "Coulple": Value Change {
        n349 = event-data() -> ()  [unwired: 1 in, 6 out]
        n350 = local read "Microscope"() -> (w703:enum16{"Miniature", "Benchtop"})
        n351 = case shown="\"AC\", 默认" "Coulple" {
          tunnel: w705 -> [w709 w724]
          tunnel: w704 -> [w708 w723]
          tunnel: w703 -> [w707 w722]
          frame "AC", Default {
            n352 = case shown="\"Benchtop\"" w707 {
              tunnel: w709 -> [w711 w717]
              tunnel: w708 -> [w710 w716]
              frame "Miniature", Default {
                n353 = xnode "读取/写入控件"("FPGA VI引用输入"=w711, "错误输入"=w710, "Adapter Module User Command"=u8 3, "Adapter Module User Data 0"=u8 0, "Adapter Module User Data 1"=u8 0, "Adapter Module Do User Command Commit"=TRUE) -> ()  [unwired: 2 out]
              }
              frame "Benchtop" {
                n354 = xnode "读取/写入控件"("FPGA VI引用输入"=w717, "错误输入"=w716, "Adapter Module User Command"=u8 3, "Adapter Module User Data 0"=u8 1, "Adapter Module User Data 1"=u8 0, "Adapter Module Do User Command Commit"=TRUE) -> ()  [unwired: 2 out]
              }
            }
          }
          frame "DC" {
            n355 = case shown="\"Benchtop\"" w722 {
              tunnel: w724 -> [w726 w732]
              tunnel: w723 -> [w725 w731]
              frame "Miniature", Default {
                n356 = xnode "读取/写入控件"("FPGA VI引用输入"=w726, "错误输入"=w725, "Adapter Module User Command"=u8 3, "Adapter Module User Data 0"=u8 0, "Adapter Module User Data 1"=u8 1, "Adapter Module Do User Command Commit"=TRUE) -> ()  [unwired: 2 out]
              }
              frame "Benchtop" {
                n357 = xnode "读取/写入控件"("FPGA VI引用输入"=w732, "错误输入"=w731, "Adapter Module User Command"=u8 3, "Adapter Module User Data 0"=u8 1, "Adapter Module User Data 1"=u8 1, "Adapter Module Do User Command Commit"=TRUE) -> ()  [unwired: 2 out]
              }
            }
          }
        }
      }
      event "Frames/Slice", "Slices": Value Change {
        n358 = event-data() -> ()  [unwired: 1 in, 6 out]
        n359 = local read "Start Dis."() -> (w740:sgl)
        n360 = local read "End Dis."() -> (w741:sgl)
        n361 = Subtract(x=w741, y=w740) -> (x-y=w739:sgl)
        n362 = Divide(x=w739, y="Slices") -> (x/y=w737:sgl)
        n363 = local write "Interval Dis."(w737) -> ()
      }
      event "Stop": Value Change {
        n364 = event-data() -> ()  [unwired: 1 in, 6 out]
      }
    }
  }
  n365 = while {
    tunnel: [w750] -> w57
    tunnel: [w749] -> w56
    tunnel: w52 -> [w748]
    tunnel: w47 -> [w747]
    stop <- w745 stop-if-true
    n366 = event shown="[0] 超时" {
      selector: _ -> [_ _]
      dyn-events: _ -> [_ _]
      timeout: 1 -> [_ _]
      tunnel: [w787 w869] -> w750
      tunnel: [w786 w868] -> w749
      tunnel: w748 -> [w789 w871]
      tunnel: w747 -> [w788 w870]
      tunnel: [_ TRUE ("FPGA Stop")] -> w745
      event Timeout {
        n367 = event-data() -> ()  [unwired: 1 in, 3 out]
        n368 = local read "Pulse Number"() -> (w769:enum16{"SP", "DP"})
        n369 = local read "Acq. Sample Rate"() -> (w759:dbl)
        n370 = Equal?(x=w769, y=enum16{"SP", "DP"}."SP") -> (x = y?=w767:bool)
        n371 = local read "Microscope"() -> (w810:enum16{"Miniature", "Benchtop"})
        n372 = case shown="\"Benchtop\"" w810 {
          tunnel: ["Zoom Miniature" "Zoom Standard"] -> w809
          frame "Miniature", Default {
          }
          frame "Benchtop" {
          }
        }
        n373 = local read "Total Data Out"() -> (w763:u16)
        n374 = Select(t=1.0, s=w767, f=2.0 ("t")) -> (s? t:f=w766:dbl)
        n375 = local read "Wave"() -> (w770:enum16{"Triangle", "Sine", "Ramp"})
        n376 = call "sub_MEMS Value to Frequency.vi"("MEMS FAST"="MEMS FAST") -> ("Ticks"=w820:u32)  [unwired: 10 in]
        n377 = call "sub_MEMS Value to Frequency.vi"("MEMS FAST"="MEMS SLOW") -> ("Ticks"=w821:u32)  [unwired: 10 in]
        n378 = case shown="0, 默认" "ZOOM" {
          selector: "ZOOM" -> [_ w861]
          tunnel: ["Y Amplitude" w859] -> w807
          tunnel: ["X Amplitude" w860] -> w812
          tunnel: w809 -> [_ w862]
          frame 0, Default {
          }
          frame 1..10 {
            n379 = Decrement(x=w861) -> (x-1=w865:u16)
            n380 = Index Array(array=w862, index (row)=w865) -> (element=w866:dbl[])  [unwired: 1 in]
            n381 = Index Array(array=w866, index #1=0 ("索引"), index #2=1 ("索引")) -> (element #1=w860:dbl, element #2=w859:dbl)  [unwired: 1 in, 1 out]
          }
        }
        n382 = local read "Line"() -> (w825:u32)
        n383 = Multiply(x="X Frequency", y=w766) -> (x*y=w827:dbl)
        n384 = Divide(x=w827, y=w825) -> (x/y=→"Frame Rate":dbl)
        n385 = call "sub_HOSTTOFPGA Voltage.vi"("Input"="Y Offset") -> ("Output"=w797:i16)
        n386 = call "sub_HOSTTOFPGA Voltage.vi"("Input"="X Offset") -> ("Output"=w762:i16)
        n387 = call "sub_HOSTTOFPGA Voltage.vi"("Input"="Laser Intensity") -> ("Output"=w794:i16)
        n388 = call "sub_HOSTTOFPGA Voltage.vi"("Input"="PMT1 Sensitivity") -> ("Output"=w801:i16)
        n389 = call "sub_HOSTTOFPGA Voltage.vi"("Input"="PMT2 Sensitivity") -> ("Output"=w780:i16)
        n390 = To Word Integer(number=w801) -> (16bit integer=w848:i16)
        n391 = case shown="\"Line Scan\"" "Scan Mode" {
          tunnel: [w852 0.0 ("数值输入控件") w854] -> w813
          tunnel: w807 -> [w852 _ w854]
          frame "Normal", Default {
          }
          frame "Line Scan" {
          }
          frame "Random Access" {
          }
        }
        n392 = To Word Integer(number=w780) -> (16bit integer=w778:i16)
        n393 = To Word Integer(number=w794) -> (16bit integer=w795:i16)
        n394 = local read "Acq. Sample Rate"() -> (w760:dbl)
        n395 = call "sub_XY Amplitude Regular.vi"("Y Amplitude"=w813, "X Amplitude"=w812) -> ("Y Amplitude Out"=w815:fxp<+,16,0>, "X Amplitude Out"=w814:fxp<+,16,0>)  [unwired: 8 in]
        n396 = local read "Wave"() -> (w774:enum16{"Triangle", "Sine", "Ramp"})
        n397 = case shown="\"SP\"" "Pulse Number" {
          tunnel: [enum16{"Single Pulse", "Two Pulse"}."Two Pulse" ("Pulse Number") enum16{"Single Pulse", "Two Pulse"}."Single Pulse" ("Pulse Number")] -> w773
          frame "DP" {
          }
          frame "SP" {
          }
        }
        n398 = call "sub_calculate value.vi"("Pixel/Line"="Pixel/Line", "Fill Fraction"="Fill Fraction", "Wave"=w774, "X Frequency"="X Frequency", "Acq. Sample Rate"=w760) -> ("Pixel Dwell"=→"Pixel Dwell":dbl, "Point/Pixel"=w757:i32)  [unwired: 5 in]
        "Point/Pixel" <- w757
        n399 = feedback #1() -> (w752:u32)  [unwired: 1 in]
        n400 = call "sub_calculate xyfrequency.vi"("Total Data Out"=w763, "Line"="Line", "Actual Output Ticks"=w752, "Actual DDS Ticks"=w752, "X Frequency"="X Frequency", "Acq. Sample Rate"=w759, "Fill Fraction"="Fill Fraction", "Back Period"="Real Back Period", "Wave"=w770) -> ("Actual DDS Sample Freq"=w793:u32, "Y Ramp Step"=w761:fxp<+/-,24,16>, "Line Out"=w791:u32, "Acq. Latch Time"=w796:u32, "Y Step"=w790:fxp<+/-,24,16>)  [unwired: 2 in]
        "Actual DDS Sample Freq" <- w793
        n401 = xnode "读取/写入控件"("FPGA VI引用输入"=w789, "错误输入"=w788, "Phase Increse"=w793, "Y Ramp Step"=w761, "Line"=w791, "Y Step"=w790, "Latch Time"=w796, "Back Period"="Real Back Period", "Laser Intensity"=w795, "X Offset"=w762, "Y Offset"=w797, "MEMS FAST"=w820, "MEMS SLOW"=w821, "PMT Sensitivity"=w848, "PMT2 Sensitivity"=w778, "X Amplitude"=w814, "Y Amplitude"=w815, "Syn. Latch Time"=u32 4 ("Latch Time"), "Pulse Number"=w773) -> ("FPGA VI引用输出"=w798:refnum<k20>, "错误输出"=w799:errorcluster, "Actual DDS Ticks"=w792:u32)
        "Actual DDS Ticks" <- w792
        n402 = feedback-in #1(w792) -> ()
        n403 = call "sub_HOSTTOFPGA Voltage.vi"("Input"="Stimulate Value") -> ("Output"=w828:i16)
        n404 = Increment(x="Frames Befor Stimulate") -> (x+1=w833:u32)
        n405 = Multiply(x="Stimulate Time", y=u32 500) -> (x*y=w835:u32)
        n406 = To Word Integer(number=w828) -> (16bit integer=w837:i16)
        n407 = xnode "读取/写入控件"("FPGA VI引用输入"=w798, "错误输入"=w799, "DDS Ticks"="DDS Ticks", "Phase Shift"="Phase Shift", "Microscope"="Microscope", "Point"="Point", "PMT1 Enable"="PMT1 Enable", "PMT2 Enable"="PMT2 Switch", "Frames Befor Stimulate"=w833, "Stimulate Interval"="Stimulate Interval", "Stimulate Time"=w835, "Stimulate Enable"="Stimulate Enable", "Vision Stimulate Value"=w837, "Wave"="Wave", "MEMS Enable"="Mems Enable", "OUTPUT Value Ticks"="OUTPUT Value Ticks", "PMT Shutter Pow."="PMT Shutter Pow.") -> ("FPGA VI引用输出"=w787:refnum<k20>, "错误输出"=w786:errorcluster, "Actual Laser Intensity"=w817:i16, "Frame Number"=w846:u32, "Stmulate Interval Dis."=→"Stimulate Time Dis.":u32, "Shock Detection"=→"Overload Dis.":bool, "Actual OUTPUT Value Ticks"=→"Actual OUTPUT Value Ticks":u32)
        n408 = call "值已改变(I32).vi"("输入数据"=w757) -> ("已更改"=w758:bool)  [unwired: 3 in]
        n409 = case shown="真" w758 {
          tunnel: w757 -> [_ w849]
          frame False {
          }
          frame True {
            n410 = property on="Point/Pixel" class="DigNum (严格)"("Val(Sgnl)"=w849) -> ()  [unwired: 2 in, 2 out]
          }
        }
        n411 = local read "Stimulate Interval"() -> (w845:u32)
        n412 = call "sub_FPGATOHOST Voltage.vi"("Input"=w817) -> ("Output"=→"Actual Laser Intensity":dbl)
        n413 = local read "Frame Rate"() -> (w844:dbl)
        n414 = Decrement(x=w846) -> (x-1=w841:u32)
        "Frame Number" <- w841
        n415 = To Double Precision Float(number=w841) -> (double precision float=w840:dbl)
        n416 = Reciprocal(x=w844) -> (1/x=w839:dbl)
        n417 = To Double Precision Float(number=w845) -> (double precision float=w842:dbl)
        n418 = Multiply(x=w840, y=w839) -> (x*y=→"Frame Befor Time":dbl)
        n419 = Multiply(x=w842, y=w839) -> (x*y=→"Stimulate Interval Time":dbl)
      }
      event "Stop": Value Change {
        n420 = event-data() -> ()  [unwired: 1 in, 3 out]
        n421 = xnode "读取/写入控件"("FPGA VI引用输入"=w871, "错误输入"=w870, "FPGA Stop"=TRUE) -> ("FPGA VI引用输出"=w873:refnum<k20>, "错误输出"=w874:errorcluster)
        n422 = xnode "Invoke Method"("FPGA VI引用输入"=w873, "错误输入"=w874) -> ("FPGA VI引用输出"=w869:refnum<k20>, "错误输出"=w868:errorcluster)
      }
    }
  }
  n423 = while {
    tunnel: w19 -> [w890]
    tunnel: w5 -> [w889]
    tunnel: [w888] -> w72
    tunnel: [w887] -> w71
    tunnel: w32 -> [w886]
    tunnel: w76 -> [w885]
    tunnel: [w884] -> w73
    tunnel: w52 -> [w881]
    tunnel: w47 -> [w880]
    border: u32 0 -> [_]
    shift-right: [w878] -> _
    shift-left: u16 0 -> [w879]
    tunnel: w21 -> [w877]
    tunnel: w22 -> [w876]
    tunnel: [w875] -> w20
    stop <- w883 stop-if-true
    # "Z-stack"
    n424 = event shown="[0] 超时" {
      selector: _ -> [_ _ _ _ _]
      dyn-events: _ -> [_ _ _ _ _]
      timeout: 1 -> [_ _ _ _ _]
      tunnel: w890 -> [w906 w993 w1098 w1238 w1265]
      tunnel: w889 -> [w905 w992 w1097 w1237 w1264]
      tunnel: [w912 w991 w1096 w1235 w1267] -> w888
      tunnel: [w908 w985 w1090 w1234 w1266] -> w887
      tunnel: w886 -> [w911 _ _ _ _]
      tunnel: w885 -> [w910 w990 w1095 w1232 w1262]
      tunnel: [w909 w990 w1095 w1232 w1262] -> w884
      tunnel: [_ _ _ _ TRUE] -> w883
      tunnel: w881 -> [_ w989 w1094 _ _]
      tunnel: w880 -> [_ w988 w1093 _ _]
      tunnel: w879 -> [w907 _ w1088 w1233 w1261]
      tunnel: [w907 u16 0 w1087 w1233 w1261] -> w878
      tunnel: w877 -> [w903 _ _ _ _]
      tunnel: w876 -> [w902 w982 w1086 w1225 w1260]
      tunnel: [w901 w982 w1086 w1225 w1260] -> w875
      event Timeout {
        n425 = event-data() -> ()  [unwired: 1 in, 3 out]
        n426 = local read "Microscope"() -> (w891:enum16{"Miniature", "Benchtop"})
        n427 = local read "Pixel/Line"() -> (w895:u16)
        n428 = local read "Line"() -> (w894:u32)
        n429 = Reciprocal(x="Acq. Start") -> (1/x=w899:dbl)
        n430 = To Fixed-Point(fixed-point type=fxp<+,18,0> 0.0, number=w899) -> (fixed-point=w898:fxp<+,18,0>)
        n431 = case shown="真" "Focus Flag" {
          tunnel: w906 -> [w920 w937]
          tunnel: w905 -> [w919 w936]
          tunnel: [w918 w944] -> w912
          tunnel: w911 -> [_ w947]
          tunnel: w910 -> [w926 w946]
          tunnel: [w926 w945] -> w909
          tunnel: [w917 w943] -> w908
          tunnel: w895 -> [_ w938]
          tunnel: w894 -> [_ w939]
          tunnel: w903 -> [_ w942]
          tunnel: w902 -> [w915 w941]
          tunnel: [w915 w940] -> w901
          frame False {
            (unwired) u32 0 ("剩余元素")
            n432 = xnode "Invoke Method"("FPGA VI引用输入"=w920, "错误输入"=w919, "元素数量"=u32 0, "超时(ms)"=0) -> ("FPGA VI引用输出"=w922:refnum<k20>, "错误输出"=w923:errorcluster, "剩余元素"=w914:u32)  [unwired: 1 out]
            n433 = Not Equal To 0?(x=w914) -> (x != 0?=w916:bool)
            n434 = local write "Rolling Queue Flag"(TRUE ("Rolling Queue Flag")) -> ()
            n435 = xnode "Invoke Method"("FPGA VI引用输入"=w922, "错误输入"=w923, "元素数量"=w914, "超时(ms)"=0) -> ("FPGA VI引用输出"=w918:refnum<k20>, "错误输出"=w917:errorcluster)  [unwired: 2 out]
            n436 = case shown="真" w916 {
              frame False {
              }
              frame True {
                n437 = feedback #2() -> (w927:u32)
                n438 = Increment(x=w927) -> (x+1=w928:u32)
                "Test Point" <- w928
                n439 = feedback-in #2(w928) -> ()
              }
            }
          }
          frame True {
            n440 = xnode "Invoke Method"("FPGA VI引用输入"=w937, "错误输入"=w936, "元素数量"=u32 0, "超时(ms)"=0) -> ("FPGA VI引用输出"=w935:refnum<k20>, "错误输出"=w934:errorcluster, "剩余元素"=w933:u32)  [unwired: 1 out]
            n441 = Multiply(x=w938, y=w939) -> (x*y=w932:u32)
            n442 = Greater Or Equal?(x=w933, y=w932) -> (x >= y?=w931:bool)
            n443 = case shown="真" w931 {
              tunnel: w947 -> [_ w971]
              tunnel: w946 -> [w949 w970]
              tunnel: [w949 w969] -> w945
              tunnel: [w951 w968] -> w944
              tunnel: [w950 w967] -> w943
              tunnel: w934 -> [w950 w966]
              tunnel: w935 -> [w951 w965]
              tunnel: w939 -> [_ w956]
              tunnel: w938 -> [_ w955]
              tunnel: w942 -> [_ w964]
              tunnel: w941 -> [w948 w963]
              tunnel: [w948 w962] -> w940
              tunnel: w932 -> [_ w961]
              frame False {
              }
              frame True {
                n444 = xnode "Invoke Method"("FPGA VI引用输入"=w965, "错误输入"=w966, "元素数量"=w961, "超时(ms)"=0) -> ("FPGA VI引用输出"=w968:refnum<k20>, "错误输出"=w967:errorcluster, "数据"=w952:fxp<+,33,17>[])  [unwired: 1 out]
                n445 = Reshape Array(w952, w956, w955) -> (w953:fxp<+,33,17>[][])
                n446 = To Unsigned Word Integer(number=w953) -> (unsigned 16bit integer=w954:u16[][])
                n447 = local read "Z-Stack"() -> (w959:bool)
                n448 = local read "Save"() -> (w958:bool)
                n449 = Enqueue Element(queue=w964, element=w954, error in (no error)=w963) -> (error out=w962:errorcluster)  [unwired: 1 in, 2 out]
                n450 = Or(x=w959, y=w958) -> (x .or. y?=w957:bool)
                n451 = case shown="真" w957 {
                  tunnel: w971 -> [_ w976]
                  tunnel: w970 -> [w972 w975]
                  tunnel: [w972 w974] -> w969
                  tunnel: w954 -> [_ w973]
                  frame False {
                  }
                  frame True {
                    n452 = Enqueue Element(queue=w976, element=w973, error in (no error)=w975) -> (error out=w974:errorcluster)  [unwired: 1 in, 2 out]
                  }
                }
              }
            }
          }
        }
        n453 = xnode "读取/写入控件"("FPGA VI引用输入"=w906, "Pixel/Line"=w895, "Line"=w894, "Microscope"=w891, "Acq.Start FXP"=w898, "Acq.Start"="Acq. Start", "Divide"="Divide") -> ("Acq. Point Dis."=→"Acq. Point Dis.":u16)  [unwired: 1 in, 2 out]
        n454 = call "sub_Acquisition Rate.vi"("Divide"="Divide") -> ("采样率"=→"Acq. Sample Rate":dbl)
      }
      event "LIVE", "Save": Value Change {
        (unwired) 0
        (unwired) u16 0
        # "高"
        # "低"
        n455 = event-data() -> ()  [unwired: 1 in, 6 out]
        n456 = local read "Save"() -> (w978:bool)
        n457 = global write "Save picture camera.vi" "Save Picture Camera"(w978) -> ()
        n458 = Compound Arithmetic op=OR ("复合运算")("LIVE", w978) -> (w980:bool)
        n459 = Build Array(w978, "LIVE") -> (w984:bool[])
        n460 = Boolean Array To Number(Boolean array=w984) -> (number=w983:u32)
        n461 = case shown="0, 默认" w983 {
          frame 1 {
            # "SAVE 1"
            # "LIVE 0"
            n462 = property on="LIVE" class="Bool (严格)"("DisabledEnum"=T4."Disabled and Grayed Out" ("禁用")) -> ()  [unwired: 2 in, 2 out]
            n463 = property on="Z-Stack" class="Bool (严格)"("DisabledEnum"=T4."Disabled and Grayed Out" ("禁用")) -> ()  [unwired: 2 in, 2 out]
          }
          frame 2 {
            # "SAVE 0"
            # "LIVE 1"
            n464 = property on="Save" class="Bool (严格)"("DisabledEnum"=T4."Disabled and Grayed Out" ("禁用")) -> ()  [unwired: 2 in, 2 out]
            n465 = property on="Z-Stack" class="Bool (严格)"("DisabledEnum"=T4."Disabled and Grayed Out" ("禁用")) -> ()  [unwired: 2 in, 2 out]
          }
          frame 0, Default {
            # "SAVE 0"
            # "LIVE 0"
            n466 = property on="Save" class="Bool (严格)"("DisabledEnum"=T4."Enabled" ("禁用")) -> ()  [unwired: 2 in, 2 out]
            n467 = property on="LIVE" class="Bool (严格)"("DisabledEnum"=T4."Enabled" ("禁用")) -> ()  [unwired: 2 in, 2 out]
            n468 = property on="Z-Stack" class="Bool (严格)"("DisabledEnum"=T4."Enabled" ("禁用")) -> ()  [unwired: 2 in, 2 out]
          }
        }
        n469 = disable-structure shown="启用" {
          disable-tunnel: [w994 _] -> w977
          frame Disabled {
            n470 = local read "Microscope"() -> (w997:enum16{"Miniature", "Benchtop"})
            n471 = Equal?(x=w997, y=enum16{"Miniature", "Benchtop"}."Benchtop") -> (x = y?=w995:bool)
            n472 = case shown="真" w995 {
              tunnel: [FALSE ("Enable") TRUE ("Enable")] -> w994
              frame False {
              }
              frame True {
              }
            }
          }
          frame Enabled {
          }
        }
        n473 = case shown="真" w980 {
          tunnel: w993 -> [w1011 w1050]
          tunnel: w992 -> [w1010 w1049]
          tunnel: [w1009 w1042] -> w991
          tunnel: [w1008 w1041] -> w986
          tunnel: w989 -> [w1007 w1048]
          tunnel: w988 -> [w1006 w1047]
          tunnel: [w1001 w1046] -> w987
          tunnel: w977 -> [w1000 w1036]
          frame False {
            n474 = flat-sequence {
              tunnel: [w1020] -> w1005
              tunnel: [w1019] -> w1004
              tunnel: [w1014] -> w1003
              tunnel: [w1013] -> w1002
              tunnel: w1011 -> [w1016]
              tunnel: w1010 -> [w1015]
              tunnel: w1007 -> [w1020]
              tunnel: w1006 -> [w1019]
              tunnel: [w1035] -> w1009
              tunnel: [w1034] -> w1008
              tunnel: [w1031] -> w1001
              tunnel: w1005 -> [w1033]
              tunnel: w1004 -> [w1032]
              tunnel: w1003 -> [w1030]
              tunnel: w1002 -> [w1029]
              tunnel: w1000 -> [_]
              frame #0 {
                n475 = local write "Focus Flag"(FALSE ("Focus Flag")) -> ()
                n476 = xnode "读取/写入控件"("FPGA VI引用输入"=w1016, "错误输入"=w1015, "FOCUS"=FALSE ("Stop Write")) -> ("FPGA VI引用输出"=w1014:refnum<k20>, "错误输出"=w1013:errorcluster)
                n477 = Wait (ms)(milliseconds to wait=u32 100 ("等待时间（毫秒）")) -> ()  [unwired: 1 out]
              }
              frame #1 {
                n478 = xnode "读取/写入控件"("FPGA VI引用输入"=w1033, "错误输入"=w1032, "Shutter"=FALSE, "Start Control"=FALSE ("Enable")) -> ("错误输出"=w1031:errorcluster)  [unwired: 1 out]
                n479 = xnode "Invoke Method"("FPGA VI引用输入"=w1030, "错误输入"=w1029, "元素数量"=u32 0, "超时(ms)"=0) -> ("FPGA VI引用输出"=w1027:refnum<k20>, "错误输出"=w1026:errorcluster, "剩余元素"=w1025:u32)  [unwired: 1 out]
                "Test Point 3" <- w1025
                n480 = xnode "Invoke Method"("FPGA VI引用输入"=w1027, "错误输入"=w1026, "元素数量"=w1025, "超时(ms)"=0) -> ("FPGA VI引用输出"=w1035:refnum<k20>, "错误输出"=w1034:errorcluster)  [unwired: 2 out]
              }
            }
          }
          frame True {
            n481 = flat-sequence {
              tunnel: w1047 -> [w1054]
              tunnel: w1048 -> [w1057]
              tunnel: w1049 -> [w1058]
              tunnel: w1050 -> [w1059]
              tunnel: [w1059] -> w1040
              tunnel: [w1058] -> w1039
              tunnel: [w1056] -> w1038
              tunnel: [w1055] -> w1037
              tunnel: w1036 -> [_]
              tunnel: [w1060] -> w1045
              tunnel: [w1063] -> w1044
              tunnel: [w1062] -> w1043
              tunnel: w1040 -> [w1063]
              tunnel: w1039 -> [w1062]
              tunnel: w1038 -> [_]
              tunnel: w1037 -> [w1060]
              tunnel: w1045 -> [w1077]
              tunnel: w1044 -> [w1072]
              tunnel: w1043 -> [w1071]
              tunnel: [w1077] -> w1046
              tunnel: [w1069] -> w1042
              tunnel: [w1068] -> w1041
              frame #0 {
                n482 = xnode "读取/写入控件"("FPGA VI引用输入"=w1057, "错误输入"=w1054, "Start Control"=TRUE ("Start"), "Shutter"=TRUE) -> ("FPGA VI引用输出"=w1056:refnum<k20>, "错误输出"=w1055:errorcluster)
                n483 = Wait (ms)(milliseconds to wait=u32 100 ("等待时间（毫秒）")) -> ()  [unwired: 1 out]
              }
              frame #1 {
                n484 = local write "Focus Flag"(TRUE ("Focus Flag")) -> ()
              }
              frame #2 {
                n485 = xnode "Invoke Method"("FPGA VI引用输入"=w1072, "错误输入"=w1071, "元素数量"=u32 0, "超时(ms)"=0) -> ("FPGA VI引用输出"=w1075:refnum<k20>, "错误输出"=w1074:errorcluster, "剩余元素"=w1073:u32)  [unwired: 1 out]
                "Test Point2" <- w1073
                n486 = xnode "Invoke Method"("FPGA VI引用输入"=w1075, "错误输入"=w1074, "元素数量"=w1073, "超时(ms)"=0) -> ("FPGA VI引用输出"=w1067:refnum<k20>, "错误输出"=w1066:errorcluster)  [unwired: 2 out]
                n487 = xnode "读取/写入控件"("FPGA VI引用输入"=w1067, "错误输入"=w1066, "FOCUS"=TRUE ("Stop Write")) -> ("FPGA VI引用输出"=w1069:refnum<k20>, "错误输出"=w1068:errorcluster)
              }
            }
          }
        }
        n488 = Merge Errors(w987, w986) -> (w985:errorcluster)
      }
      event "Z-Stack": Value Change {
        n489 = event-data() -> ()  [unwired: 1 in, 6 out]
        n490 = disable-structure shown="禁用" {
          disable-tunnel: [w1099 _] -> w1085
          frame Disabled {
            n491 = local read "Microscope"() -> (w1100:enum16{"Miniature", "Benchtop"})
            n492 = Equal?(x=w1100, y=enum16{"Miniature", "Benchtop"}."Benchtop") -> (x = y?=w1102:bool)
            n493 = case shown="假" w1102 {
              tunnel: [FALSE ("Enable") TRUE ("Enable")] -> w1099
              frame False {
              }
              frame True {
              }
            }
          }
          frame Enabled {
          }
        }
        n494 = case shown="真" "Z-Stack" {
          tunnel: w1098 -> [w1123 w1194]
          tunnel: w1097 -> [w1122 w1193]
          tunnel: [w1121 w1186] -> w1096
          tunnel: [w1120 w1185] -> w1091
          tunnel: w1094 -> [w1119 w1192]
          tunnel: w1093 -> [w1118 w1191]
          tunnel: [w1113 w1190] -> w1092
          tunnel: w1088 -> [w1109 w1177]
          tunnel: [w1106 w1180] -> w1087
          tunnel: w1085 -> [_ w1176]
          frame False {
            n495 = flat-sequence {
              tunnel: [w1133] -> w1117
              tunnel: [w1132] -> w1116
              tunnel: [w1127] -> w1115
              tunnel: [w1126] -> w1114
              tunnel: w1123 -> [w1129]
              tunnel: w1122 -> [w1128]
              tunnel: w1119 -> [w1133]
              tunnel: w1118 -> [w1132]
              tunnel: w1109 -> [w1124]
              tunnel: [w1124] -> w1108
              tunnel: w1117 -> [w1147]
              tunnel: w1116 -> [w1146]
              tunnel: w1115 -> [w1144]
              tunnel: w1114 -> [w1143]
              tunnel: [w1149] -> w1112
              tunnel: [w1148] -> w1111
              tunnel: [w1145] -> w1110
              tunnel: w1108 -> [w1135]
              tunnel: [w1135] -> w1107
              tunnel: [w1134] -> w1105
              tunnel: [w1151] -> w1113
              tunnel: [w1155] -> w1120
              tunnel: [w1157] -> w1121
              tunnel: w1112 -> [w1156]
              tunnel: w1111 -> [w1154]
              tunnel: w1110 -> [w1152]
              tunnel: w1107 -> [w1161]
              tunnel: [w1159] -> w1106
              tunnel: w1105 -> [w1153]
              frame #0 {
                n496 = local write "Focus Flag"(FALSE ("Focus Flag")) -> ()
                n497 = xnode "读取/写入控件"("FPGA VI引用输入"=w1129, "错误输入"=w1128, "FOCUS"=FALSE ("Stop Write")) -> ("FPGA VI引用输出"=w1127:refnum<k20>, "错误输出"=w1126:errorcluster)
                n498 = Wait (ms)(milliseconds to wait=u32 50 ("等待时间（毫秒）")) -> ()  [unwired: 1 out]
              }
              frame #1 {
                n499 = xnode "Invoke Method"("FPGA VI引用输入"=w1144, "错误输入"=w1143, "元素数量"=u32 0, "超时(ms)"=0) -> ("FPGA VI引用输出"=w1141:refnum<k20>, "错误输出"=w1140:errorcluster, "剩余元素"=w1139:u32)  [unwired: 1 out]
                n500 = xnode "读取/写入控件"("FPGA VI引用输入"=w1147, "错误输入"=w1146, "Start Control"=FALSE ("Enable")) -> ("FPGA VI引用输出"=w1134:refnum<k20>, "错误输出"=w1145:errorcluster)
                n501 = xnode "Invoke Method"("FPGA VI引用输入"=w1141, "错误输入"=w1140, "元素数量"=w1139, "超时(ms)"=0) -> ("FPGA VI引用输出"=w1149:refnum<k20>, "错误输出"=w1148:errorcluster)  [unwired: 2 out]
              }
              frame #2 {
                n502 = local read "Slices"() -> (w1150:u16)
                n503 = Increment(x=w1161) -> (x+1=w1158:u16)
                n504 = Greater Or Equal?(x=w1158, y=w1150) -> (x >= y?=w1160:bool)
                n505 = case shown="假" w1160 {
                  tunnel: [w1165 u16 0] -> w1159
                  tunnel: w1158 -> [w1165 _]
                  tunnel: [w1164 w1171] -> w1157
                  tunnel: w1156 -> [w1164 w1171]
                  tunnel: [w1163 w1172] -> w1155
                  tunnel: w1154 -> [w1163 w1172]
                  tunnel: w1153 -> [_ w1169]
                  tunnel: w1152 -> [w1162 w1168]
                  tunnel: [w1162 w1167] -> w1151
                  frame False {
                    n506 = property on="Move" class="Bool (严格)"("Val(Sgnl)"=TRUE ("值(信号)")) -> ()  [unwired: 2 in, 2 out]
                  }
                  frame True {
                    n507 = xnode "读取/写入控件"("FPGA VI引用输入"=w1169, "错误输入"=w1168, "Shutter"=FALSE ("Enable")) -> ("错误输出"=w1167:errorcluster)  [unwired: 1 out]
                    n508 = property on="Save" class="Bool (严格)"("DisabledEnum"=T4."Enabled" ("禁用")) -> ()  [unwired: 2 in, 2 out]
                    n509 = property on="LIVE" class="Bool (严格)"("DisabledEnum"=T4."Enabled" ("禁用")) -> ()  [unwired: 2 in, 2 out]
                  }
                }
              }
            }
          }
          frame True {
            n510 = flat-sequence {
              tunnel: w1191 -> [w1198]
              tunnel: w1192 -> [w1201]
              tunnel: w1193 -> [w1202]
              tunnel: w1194 -> [w1203]
              tunnel: [w1203] -> w1184
              tunnel: [w1202] -> w1183
              tunnel: [w1200] -> w1182
              tunnel: [w1199] -> w1181
              tunnel: [w1197] -> w1178
              tunnel: w1177 -> [w1197]
              tunnel: w1176 -> [_]
              tunnel: [w1205] -> w1189
              tunnel: [w1208] -> w1188
              tunnel: [w1207] -> w1187
              tunnel: w1184 -> [w1208]
              tunnel: w1183 -> [w1207]
              tunnel: w1182 -> [_]
              tunnel: w1181 -> [w1205]
              tunnel: [w1204] -> w1179
              tunnel: w1178 -> [w1204]
              tunnel: w1189 -> [w1223]
              tunnel: w1188 -> [w1218]
              tunnel: w1187 -> [w1217]
              tunnel: [w1223] -> w1190
              tunnel: [w1215] -> w1186
              tunnel: [w1214] -> w1185
              tunnel: [w1209] -> w1180
              tunnel: w1179 -> [w1209]
              frame #0 {
                w1195 = TRUE ("Start")
                n511 = xnode "读取/写入控件"("FPGA VI引用输入"=w1201, "错误输入"=w1198, "Start Control"=w1195, "Shutter"=w1195) -> ("FPGA VI引用输出"=w1200:refnum<k20>, "错误输出"=w1199:errorcluster)
                n512 = Wait (ms)(milliseconds to wait="Interval Time") -> ()  [unwired: 1 out]
              }
              frame #1 {
                n513 = local write "Focus Flag"(TRUE ("Focus Flag")) -> ()
              }
              frame #2 {
                n514 = xnode "Invoke Method"("FPGA VI引用输入"=w1218, "错误输入"=w1217, "元素数量"=u32 0, "超时(ms)"=0) -> ("FPGA VI引用输出"=w1221:refnum<k20>, "错误输出"=w1220:errorcluster, "剩余元素"=w1219:u32)  [unwired: 1 out]
                n515 = xnode "Invoke Method"("FPGA VI引用输入"=w1221, "错误输入"=w1220, "元素数量"=w1219, "超时(ms)"=0) -> ("FPGA VI引用输出"=w1213:refnum<k20>, "错误输出"=w1212:errorcluster)  [unwired: 2 out]
                n516 = xnode "读取/写入控件"("FPGA VI引用输入"=w1213, "错误输入"=w1212, "FOCUS"=TRUE ("Stop Write")) -> ("FPGA VI引用输出"=w1215:refnum<k20>, "错误输出"=w1214:errorcluster)
              }
            }
          }
        }
        n517 = case shown="真" "Z-Stack" {
          frame False {
          }
          frame True {
          }
        }
        n518 = Merge Errors(w1092, w1091) -> (w1090:errorcluster)
      }
      event "Pixel/Line", "Line": Value Change {
        n519 = event-data() -> ()  [unwired: 1 in, 6 out]
        n520 = xnode "读取/写入控件"("FPGA VI引用输入"=w1238, "错误输入"=w1237, "FOCUS"=FALSE) -> ("FPGA VI引用输出"=w1231:refnum<k20>, "错误输出"=w1228:errorcluster)
        n521 = flat-sequence {
          tunnel: w1231 -> [w1253]
          tunnel: [w1253] -> w1230
          tunnel: [w1252] -> w1229
          tunnel: w1228 -> [w1252]
          frame #0 {
            n522 = Wait (ms)(milliseconds to wait=u32 5 ("等待时间（毫秒）")) -> ()  [unwired: 1 out]
          }
        }
        n523 = xnode "Invoke Method"("FPGA VI引用输入"=w1230, "错误输入"=w1229, "元素数量"=u32 0, "超时(ms)"=0) -> ("FPGA VI引用输出"=w1241:refnum<k20>, "错误输出"=w1242:errorcluster, "剩余元素"=w1239:u32)  [unwired: 1 out]
        n524 = xnode "Invoke Method"("FPGA VI引用输入"=w1241, "错误输入"=w1242, "元素数量"=w1239, "超时(ms)"=0) -> ("FPGA VI引用输出"=w1227:refnum<k20>, "错误输出"=w1226:errorcluster)  [unwired: 2 out]
        n525 = local read "LIVE"() -> (w1224:bool)
        n526 = case shown="假" w1224 {
          tunnel: [w1246 w1250] -> w1235
          tunnel: [w1245 w1249] -> w1234
          tunnel: w1227 -> [w1246 w1248]
          tunnel: w1226 -> [w1245 w1247]
          frame False {
          }
          frame True {
            n527 = xnode "读取/写入控件"("FPGA VI引用输入"=w1248, "错误输入"=w1247, "FOCUS"=TRUE) -> ("FPGA VI引用输出"=w1250:refnum<k20>, "错误输出"=w1249:errorcluster)
          }
        }
      }
      event "Stop": Value Change {
        n528 = event-data() -> ()  [unwired: 1 in, 3 out]
        n529 = xnode "Invoke Method"("FPGA VI引用输入"=w1265, "错误输入"=w1264) -> ("FPGA VI引用输出"=w1259:refnum<k20>, "错误输出"=w1258:errorcluster)
        n530 = xnode "Invoke Method"("FPGA VI引用输入"=w1259, "错误输入"=w1258) -> ("FPGA VI引用输出"=w1257:refnum<k20>, "错误输出"=w1256:errorcluster)
        n531 = xnode "Invoke Method"("FPGA VI引用输入"=w1257, "错误输入"=w1256) -> ("FPGA VI引用输出"=w1267:refnum<k20>, "错误输出"=w1266:errorcluster)
        "Power Stop" <- TRUE ("Power Stop")
      }
    }
  }
  n532 = local read "Rolling Average"() -> (w33:dbl)
  n533 = Obtain Queue(max queue size (-1, unlimited)=w33, name (unnamed)="Rolling Init" ("名称（未命名）"), element data type=dbl[][] [] ("x/y")) -> (queue out=w45:refnum<queue>, error out=w46:errorcluster)  [unwired: 2 in, 1 out]
  n534 = call "IMAQ Create"("Image Name"="ROI Mask", "Image Type"=w3) -> ("New Image"=w2:T1, "error out"=w1:errorcluster)  [unwired: 3 in]
  n535 = call "IMAQ Create"("Image Name"="Rolling", "Image Type"=w35) -> ("New Image"=w39:T1)  [unwired: 3 in, 1 out]
  n536 = call "IMAQ Create"("Image Name"="Display-IMAQ", "Image Type"=w9) -> ("New Image"=w8:T1)  [unwired: 3 in, 1 out]
  n537 = call "IMAQ Create"("Image Name"="92", "Image Type"=w15) -> ("New Image"=w13:T1, "error out"=w12:errorcluster)  [unwired: 3 in]
  n538 = Initialize Array(0.0 ("元素"), w38, w38) -> (w36:dbl[][])
  n539 = while {
    shift-right: [w1285] -> _
    shift-left: w36 -> [w1286]
    tunnel: w39 -> [w1284]
    shift-right: [w1283] -> w40
    shift-left: w45 -> [w1281]
    shift-right: [w1282] -> w41
    shift-left: w46 -> [w1280]
    shift-right: [w1279] -> _
    shift-left: 1.0 ("Rolling Average") -> [w1278]
    tunnel: w21 -> [w1276]
    shift-right: [w1273] -> _
    shift-left: u16 0 -> [w1274]
    tunnel: w13 -> [w1272]
    tunnel: w12 -> [w1271]
    tunnel: w8 -> [w1270]
    tunnel: w2 -> [w1269]
    tunnel: w1 -> [w1268]
    i -> [w1277]
    stop <- w1289 stop-if-true
    n540 = Dequeue Element(queue=w1276) -> (queue out=w1275:refnum<queue>, element=w1287:u16[][], error out=w1288:errorcluster)  [unwired: 2 in, 1 out]
    n541 = case shown="无错误" w1288 {
      tunnel: [_ TRUE] -> w1289
      tunnel: w1287 -> [w1292 _]
      tunnel: w1286 -> [w1311 _]
      tunnel: [w1297 dbl[][] [] ("x/y")] -> w1285
      tunnel: w1284 -> [w1306 _]
      tunnel: [w1316 w1417] -> w1283
      tunnel: [w1309 w1416] -> w1282
      tunnel: w1281 -> [w1314 w1417]
      tunnel: w1280 -> [w1313 w1416]
      tunnel: [w1312 w1415] -> w1279
      tunnel: w1278 -> [w1315 w1415]
      tunnel: w1277 -> [w1310 _]
      tunnel: w1275 -> [w1308 _]
      tunnel: w1274 -> [w1304 _]
      tunnel: [w1303 u16 0] -> w1273
      tunnel: w1272 -> [w1301 _]
      tunnel: w1271 -> [w1300 _]
      tunnel: w1270 -> [w1298 _]
      tunnel: w1269 -> [w1295 _]
      tunnel: w1268 -> [w1293 _]
      frame No Error {
        n542 = local read "Pulse Number"() -> (w1291:enum16{"SP", "DP"})
        n543 = Get Queue Status(queue=w1308) -> (# elements in queue=→"Memory":i32)  [unwired: 2 in, 7 out]
        n544 = Increment(x=w1304) -> (x+1=w1303:u16)
        "Total Frames" <- w1303
        n545 = call "sub_bidirection重组.vi"("Pulse Number"=w1291, "Input"=w1292) -> ("合并数组"=w1290:u16[][][])  [unwired: 1 in, 2 out]
        n546 = Subtract(x=u16 65535, y=w1290) -> (x-y=w1299:u16[][][])
        n547 = case shown="真" "Rolling" {
          tunnel: [w1356 w1378] -> w1297
          tunnel: [w1355 w1377] -> w1316
          tunnel: w1315 -> [w1354 _]
          tunnel: w1314 -> [w1355 w1376]
          tunnel: w1313 -> [w1358 w1375]
          tunnel: [w1354 w1374] -> w1312
          tunnel: w1311 -> [w1356 w1373]
          tunnel: w1310 -> [_ w1372]
          tunnel: [w1357 w1371] -> w1309
          tunnel: w1299 -> [w1360 w1370]
          tunnel: w1306 -> [_ w1369]
          tunnel: [w1359 w1367] -> w1296
          tunnel: w1298 -> [w1353 _]
          frame False {
            n548 = for {
              tunnel: w1360 -> [w1365] mode=indexing
              shift-right: [w1362] -> w1357
              shift-left: w1358 -> [w1363]
              shift-right: [w1364] -> w1359
              shift-left: w1353 -> [w1361]
              n549 = call "IMAQ ArrayToImage"("Image Pixels (U16)"=w1365, "error in (no error)"=w1363, "Image"=w1361) -> ("error out"=w1362:errorcluster, "Image Out"=w1364:T1)  [unwired: 7 in]
            }
          }
          frame True {
            n550 = for {
              tunnel: [w1395] -> w1378
              tunnel: w1373 -> [w1390]
              tunnel: w1372 -> [w1389]
              tunnel: w1370 -> [w1387] mode=indexing
              tunnel: "Rolling Queue Flag" -> [w1379]
              shift-right: [w1394] -> w1377
              shift-left: w1376 -> [w1393]
              shift-right: [w1388] -> w1371
              shift-left: w1375 -> [w1392]
              shift-right: [w1380] -> w1367
              shift-left: w1369 -> [w1386]
              shift-right: [w1391] -> w1374
              shift-left: "Rolling Average" -> [w1382]
              n551 = case shown="真" w1379 {
                tunnel: [w1399 w1405] -> w1383
                tunnel: [w1397 w1404] -> w1385
                tunnel: [w1398 w1412] -> w1391
                tunnel: w1382 -> [w1398 w1412]
                tunnel: w1393 -> [w1399 w1407]
                tunnel: w1392 -> [w1397 w1406]
                tunnel: [w1396 w1409] -> w1384
                tunnel: w1390 -> [w1396 _]
                tunnel: w1389 -> [_ w1401]
                frame False {
                }
                frame True {
                  w1410 = 2048 ("维数大小")
                  n552 = Release Queue(queue=w1407, error in (no error)=w1406) -> ()  [unwired: 1 in, 3 out]
                  n553 = local write "Rolling Queue Flag"(FALSE ("Rolling Queue Flag")) -> ()
                  n554 = Number To Decimal String(number=w1401) -> (decimal integer string=w1402:string)  [unwired: 1 in]
                  n555 = Obtain Queue(max queue size (-1, unlimited)=w1412, name (unnamed)=w1402, element data type=dbl[][] [] ("x/y")) -> (queue out=w1408:refnum<queue>, error out=w1403:errorcluster)  [unwired: 2 in, 1 out]
                  n556 = Initialize Array(0.0 ("元素"), w1410, w1410) -> (w1409:dbl[][])
                  n557 = Flush Queue(queue=w1408, error in (no error)=w1403) -> (queue out=w1405:refnum<queue>, error out=w1404:errorcluster)  [unwired: 1 out]
                }
              }
              n558 = call "sub_rolling average.vi"("Raw Data"=w1387, "错误输入（无错误）"=w1385, "队列输入"=w1383, "移位in"=w1384, "Image Create"=w1386) -> ("错误输出"=w1388:errorcluster, "队列输出"=w1394:refnum<queue>, "移位out"=w1395:dbl[][], "Image Display"=w1380:T1, "队列中元素数量"=→"Queue Number":i32)  [unwired: 2 in]
            }
          }
        }
        "Image" <- w1296
        n559 = case shown="真" "ROI Statistic" {
          tunnel: w1296 -> [_ w1322]
          tunnel: w1295 -> [_ w1323]
          tunnel: w1293 -> [_ w1321]
          frame False {
          }
          frame True {
            n560 = property on="Image" class="ImageControl"() -> ("ROI"=w1324:T5)  [unwired: 2 in, 2 out]
            n561 = call "ROI统计量16bit.vi"("error in (no error)"=w1321, "ROI Descriptor"=w1324, "Image Mask"=w1323, "Image"=w1322) -> ("统计量"=w1325:sgl[])  [unwired: 5 in, 2 out]
            n562 = Index Array(array=w1325, index #1=0 ("索引"), index #2=1 ("索引"), index #3=2 ("索引"), index #4=3 ("索引")) -> (element #1=w1319:sgl, element #2=→"Variation":sgl, element #3=→"Minimal":sgl, element #4=→"Maximal":sgl)
            n563 = Subtract(x=w1319, y=sgl 32751.0) -> (x-y=→"Mean Value" →"波形图表":sgl)
          }
        }
        n564 = disable-structure shown="启用" {
          disable-tunnel: "Calculate Phase shift" -> [w1336 _]
          disable-tunnel: w1296 -> [w1335 _]
          disable-tunnel: w1301 -> [w1334 _]
          disable-tunnel: w1300 -> [w1333 _]
          frame Enabled {
            n565 = case shown="真" w1336 {
              tunnel: w1335 -> [_ w1339]
              tunnel: w1334 -> [_ w1338]
              tunnel: w1333 -> [_ w1337]
              frame False {
              }
              frame True {
                n566 = property on="Image" class="ImageControl"() -> ("ROI"=w1342:T5)  [unwired: 2 in, 2 out]
                n567 = Unbundle By Name(w1342) -> ("Global Rectangle"=w1344:i32[])
                n568 = call "sub_转换成偶数数组.vi"("输入数组"=w1344) -> ("输出数组"=w1343:i32[])
                n569 = call "IMAQ Extract 2"("Optional Rectangle"=w1343, "error in (no error)"=w1337, "Image Dst"=w1338, "Image Src"=w1339) -> ("error out"=w1347:errorcluster, "Image Dst Out"=w1346:T1)  [unwired: 6 in]
                n570 = call "IMAQ ImageToArray"("error in (no error)"=w1347, "Image"=w1346) -> ("Image Pixels (U16)"=w1345:u16[][])  [unwired: 2 in, 4 out]
                n571 = To Double Precision Float(number=w1345) -> (double precision float=w1348:dbl[][])
                n572 = Subtract(x=w1348, y=32768.0) -> (x-y=w1350:dbl[][])
                n573 = call "sub_提取奇偶行2.vi"("数组"=w1350) -> ("奇数行一维数组"=w1352:dbl[], "偶数行一维数组"=w1351:dbl[])  [unwired: 5 in]
                n574 = call "sub_互相关.vi"("互相关点数"="互相关点数", "y"=w1351, "x"=w1352) -> ("中心偏移"=→"中心偏移":i32)  [unwired: 2 in, 2 out]
              }
            }
          }
          frame Disabled {
          }
        }
      }
      frame Error {
      }
    }
  }
  n575 = xnode "关闭FPGA VI引用"("FPGA VI引用输入"=w57, "错误输入"=w56) -> ()  [unwired: 1 out]
  n576 = Release Queue(queue=w32, error in (no error)=w73) -> ()  [unwired: 1 in, 3 out]
  n577 = Release Queue(queue=w21, error in (no error)=w20) -> ()  [unwired: 1 in, 3 out]
  n578 = Release Queue(queue=w40, error in (no error)=w41) -> ()  [unwired: 1 in, 3 out]
  n579 = xnode "关闭FPGA VI引用"("FPGA VI引用输入"=w72, "错误输入"=w71) -> ()  [unwired: 1 out]
